vi "Measurement.vi"(0 "Position":T7(array[cluster]) {"Z" format="%.1f"; "Y" format="%.1f"; "X" format="%.1f"}, 1 "setup":T8=enum."Show Setup", 2 "Post Process":T5, 4 "File":T9, 5 "Results file":path, 7 "Raw data file":path, 11 "Setup filename":string) -> (14 "2nd plot":cluster{"Xo":dbl, "Delta X":dbl, dbl[]}[](graph), 19 "Status Out":T4)   [LabVIEW 2010]
uses:
  Anemometry Sub Vis/Controls/Save_Data.ctl
  Anemometry Sub Vis/Controls/Setup.ctl
  Anemometry Sub Vis/Controls/Graph_Type.ctl
  Anemometry Sub Vis/Controls/Post_Process.ctl
  Anemometry Sub Vis/Gen Trav/Multi_Run_Status.ctl
  Anemometry Sub Vis/Controls/Board_Types.ctl
  Anemometry Sub Vis/File/Setup_Filetype.ctl
  Anemometry Sub Vis/Controls/Block_start_and_end.ctl
  ADAM Client/Sub VIs/ADAM Controls/Traverse_Level_State.ctl
  Anemometry Sub Vis/Globals/Trav_pos_global.vi
  Anemometry Sub Vis/Globals/Meas_global.vi
  Anemometry Sub Vis/Acquisition/Data_Translation/DataTranslation_global.vi
  Anemometry Sub Vis/Acquisition/PWA/PWAtasksGLOBAL.vi
  Anemometry Sub Vis/Globals/Preference_global.vi
  Anemometry Sub Vis/Globals/LDA_meas_global_1.vi
  Anemometry Sub Vis/Globals/Dynamic_call_global.ph.vi
  Anemometry Sub Vis/Globals/LDA_meas_global_2.vi
  Anemometry Sub Vis/Globals/Plug_in_data_global.vi
panel:
  in  "PP next block":bool
  out "Pause message":string
  out "Statistics":string[][](table)
  in  "Tab Control":T1(tab)
  out "Measurement time (min)":dbl=6.0 format="%.2f"
  in  "No of bins":i32=80
  in  "Show Smoth":bool=TRUE
  in  "Second Graph":T3={"Plot 1"=2, "Plot 2"=1, "Save graph"=0, "Plot Type"=enum."Vel histogram"} {"Save graph" items=["Do not save plot", "Save plot"]; "Plot 2" items=["Nothing", "Pitot (C)"]; "Plot 1" items=["Nothing", "Pitot (C)"]}
  in  "First Graph":T3={"Plot 1"=1, "Plot 2"=2, "Save graph"=0, "Plot Type"=enum."Velocity trace"} {"Save graph" items=["Do not save plot", "Save plot"]; "Plot 2" items=["Nothing", "Pitot (C)"]; "Plot 1" items=["Nothing", "Pitot (C)"]}
  out "First plot":cluster{"Xo":dbl, "Delta X":dbl, dbl[]}[](graph)
  in  "Comments":string
  out "BSA Diagnostic info":string[][](table)
  out "uv":dbl[][](graph)=[[-0.041806189081711534, -0.046435429052714985, -0.04035660097427599, -0.042187605126076694, -0.042052555599004206]]
  out "u^4":dbl[][](graph)
  out "u^3":dbl[][](graph)
  out "u^2":dbl[][](graph)=[[0.09743628875280319, 0.10575821456272283, 0.10126262927293661, 0.09890442087602569, 0.1022948212436432]]
  out "U":dbl[][](graph)=[[0.8295029456391334, 0.8915896983798417, 0.8415763502225625, 0.8394746126219594, 0.8466062785395404]]
  in  "Block average display control":cluster{"Name":string, "Include":bool}[](array[cluster])=[{"Name"="FF (C)", "Include"=FALSE}]
  out "Array U":dbl[][](array[numeric]) format="%.2e"
  out "Array u^2":dbl[][](array[numeric]) format="%.2e"
  out "Actual Sampling freq":dbl=100.0 format="%.1f"
  in  "Desired Sampling freq (Hz)":dbl=100.0 format="%.1f"
  in  "Correlate?":T6(ring)
  out "Current Block No":i32=5
  in  "Pause":bool
  in  "No of Blocks":i32=5
  in  "stop":bool
  in  "No of samples":i32=1000 min=0 step=1
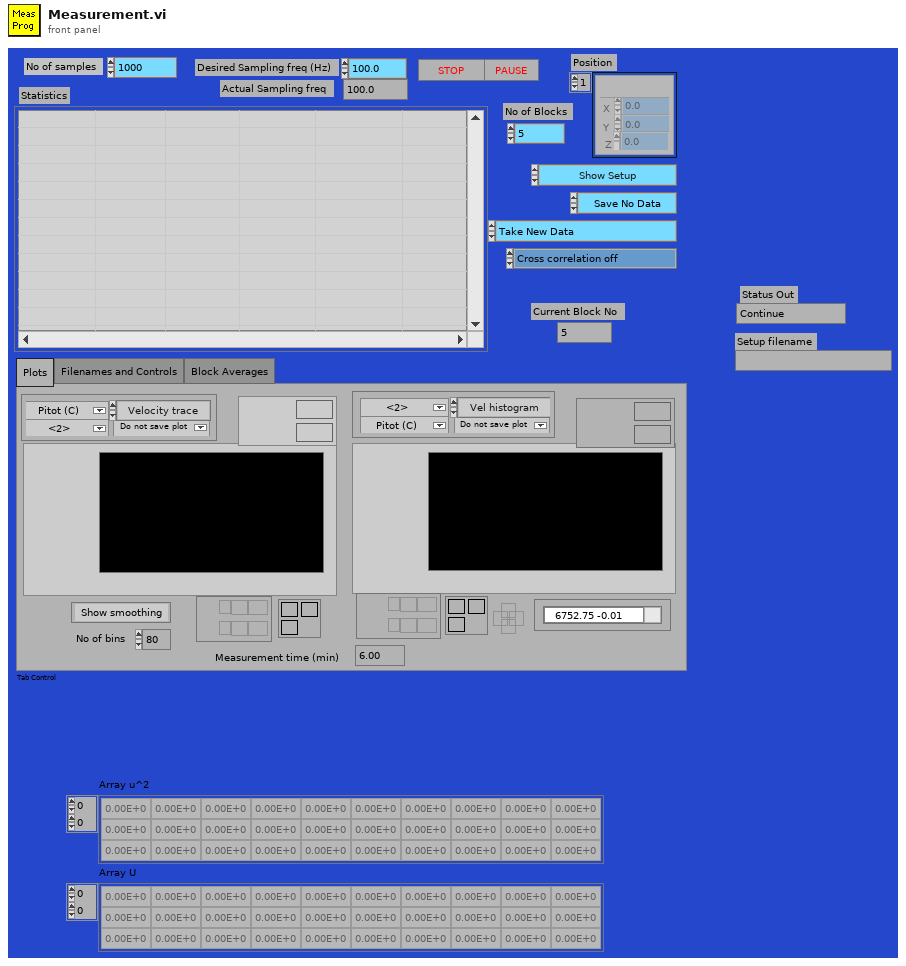
[diagram p1: front panel]
types:
  T1 = enum32{"Plots", "Filenames and Controls", "Block Averages"}
  T2 = typedef "Graph_Type.ctl" = enum16{"Show no graph", "Voltage trace", "Velocity trace", "Vel histogram", "Spectrum", "f.E(f) v Log f", "Auto-Corr"}
  T3 = cluster{"Plot 1":u16, "Plot 2":u16, "Save graph":u16, "Plot Type":T2}
  T4 = typedef "Multi_Run_Status.ctl" = enum16{"Continue", "Jump to Next Point", "Jump to Next Row", "Jump To Fall Back", "Terminate Run"}
  T5 = typedef "Post_Process.ctl" = enum16{"Take New Data", "Post Process Raw Data File"}
  T6 = enum16{"Cross correlation off", "Show correlation panel", "Correlate without activating panel"}
  T7 = cluster{"Name":string, "X":dbl, "Y":dbl, "Z":dbl}[]
  T8 = typedef "Setup.ctl" = enum16{"Run Program", "Show Setup", "Save Current Setup", "Setup Front Panel"}
  T9 = typedef "Save_Data.ctl" = enum16{"Save No Data", "Save Data"}
  T10 = enum32{"Bad", "Idle", "Run top level", "Running"}
  T11 = enum16{"Velocity", "Transit time", "Arrival time"}
  T12 = enum16{"Save no data", "Save data in new files", "Save data in existing files"}
  T13 = typedef "Board_Types.ctl" = enum16{"Simulate", "Local ADAM", "Server ADAM", "NI-DAQmx", "NI-DAQmxBase", "ADC488", "DT LV-link"}
  T14 = typedef "Setup_Filetype.ctl" = enum16{"Measurement Setups", "Calibration Setups", "General", "Results File Plotter Setups", "Speed Calib Tweaks"}
  T15 = typedef "Block_start_and_end.ctl" = cluster{"Started":dbl, "Ended":dbl, "Analogue Frequency Hz":dbl}
  T16 = typedef "Traverse_Level_State.ctl" = enum16{"Running", "Complete"}
  T17 = typedef "Traverse_cluster.ctl" = cluster{"Start X":dbl, "Start Y":dbl, "Start Z":dbl, "End X":dbl, "End Y":dbl, "End Z":dbl, "No. of pts.":i32, "Spacing":T18, "Filename":path, "Tunnel Speed":dbl, "Averaging time (min)":dbl, "Extra Commands":string, "Specific Arguments":string, "Emission Rate (l/min)":dbl, "Trace Gas Concentration (%)":dbl, "Density Ratio":string, "Comments":string, "Row No":i32, "Row Type Selector":T19, "Completion time":string, "Row Duration (mins)":dbl, "No. of Valid pts.":i32, "Meas Setup File":string}
  T18 = typedef "Spacing.ctl" = enum16{"Linear", "Log", "Gauss", "Specified", "N/A"}
  T19 = typedef "Multi_run_mode.ctl" = enum16{"Move Traverse Only", "Set Tunnel Speed Only", "Set Source Only", "Set Measurement Conditions", "Single Measurement", "Vertical Profile", "Lateral Profile", "Longitudinal Profile", "Explore Volume", "Multi-Axis Profile", "Auto Calibrate", "Meas Fast FID Bkgnd", "Check Beam Power", "Scanning Valve Measurement", "Run VI Named:", "Set ADAM Ch", "Wait (minutes)", "Send Message", "Synchronize With:", "Fall Back to this Row", "Turn Off Row Repeating", "Blank Row"}
  T20 = typedef "Analysis_info_cluster.ctl" = cluster{"Colour":u32, "Inst type":T21, "Inst name":string, "Symbol":string, "Code name":string, "Extra Info":string, "Inst Array":T22, "Index":i32, "Voltage Index":i32, "Extra Titles":string[], "Extra Values":string[]}
  T21 = typedef "Inst_type.ctl" = enum16{"Propeller anemometer", "Raw voltage", "Pressure Transducer", "Pitot-static tube", "Preston tube", "Hot wire", "Cross wire 1", "Cross wire 2", "Generic Linear", "Generic Polynomial", "Generic BackPoly", "Fast FID", "Thermocouple", "Cold wire", "Pulsed Wire", "LDA Vel", "LDA Tran time", "LDA Arr time"}
  T22 = typedef "Instrument_Array.ctl" = enum16{"PWA", "LDA", "Analogue"}
  T23 = enum16{"Velocity", "Transit time", "Arrival time"}[]
  T24 = typedef "BSA_Type.ctl" = enum16{"57N11", "BSA F60"}
  T25 = typedef "BSA_info_Cluster.ctl" = cluster{"GPIB Address":string, "No of Check Bytes":i32, "Extra Info":string, "COLOUR":u32, "Wavelength (nm)":dbl}
  T26 = typedef "Ch_and_Spans.ctl" = cluster{"high limit (10V)":sgl, "low limit (-10V)":sgl, "Ch No":i16, "Var name":string, "Use Latest Calib":bool}
  T27 = typedef "Velocity_cluster.ctl" = cluster{"Name":string, "U":dbl, "u^2":dbl, "u^3/(u^2)^(1.5)":dbl, "u^4/(u^2)^2 -3":dbl, "% u'/U":dbl, "Mean % Err":dbl, "u^4":dbl}
  T28 = typedef "Analysis_type_cluster.ctl" = cluster{"Analysis type":T29, "Indicies":i32[], "Name":string, "Inst Array":T22, "Info index":i32}
  T29 = typedef "Analysis_type_Enum.ctl" = enum16{"Slow Response", "Fast Response", "Weighted Fast Response", "Fast FID", "Weighted Fast FID", "Cross Wire", "Weighted Cross Wire", "Weighted LDA"}
  T30 = cluster{"Insts for plotting[0]":u16, "Insts for plotting[1]":u16}
  T31 = typedef "PWA_Data.ctl" = enum16{"No PWA Data", "One Ch PWA"}
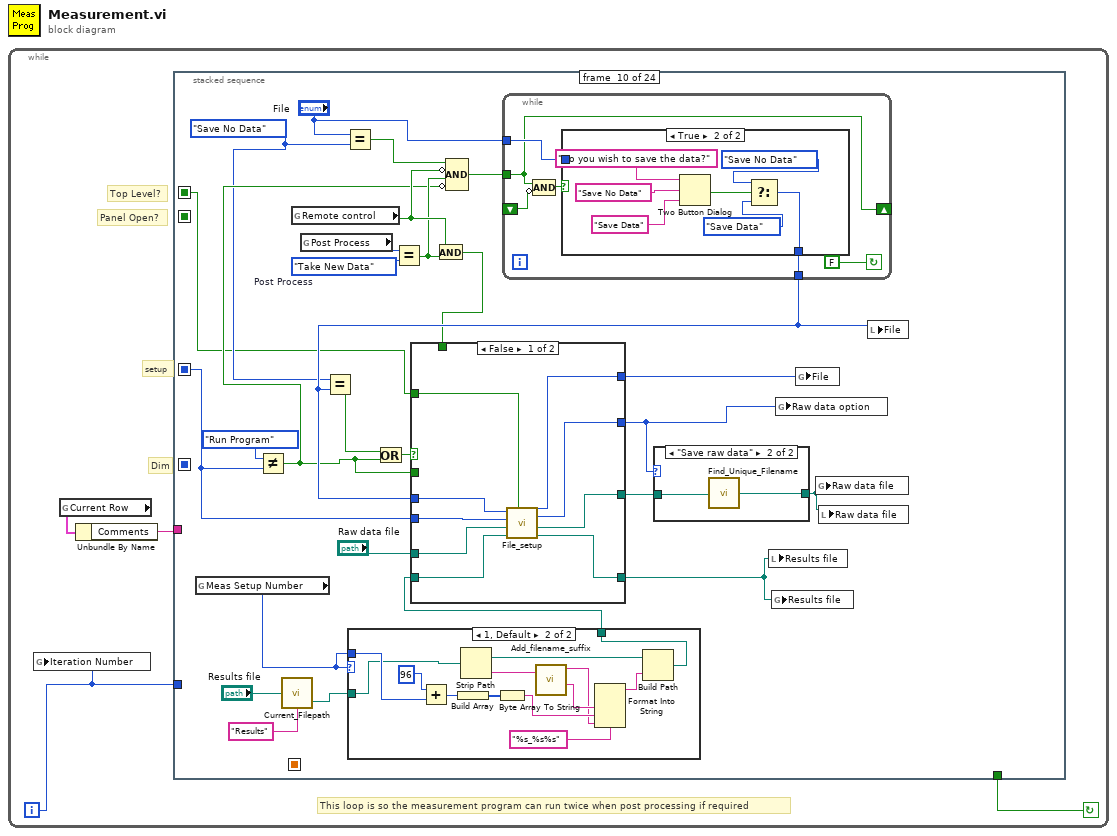
[diagram p0: block diagram]
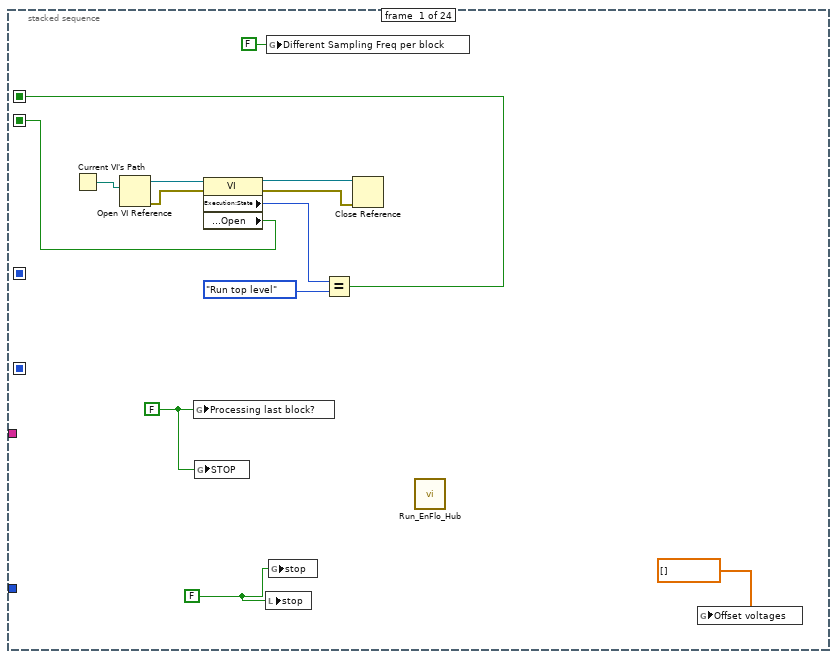
[diagram p2: hidden frame]
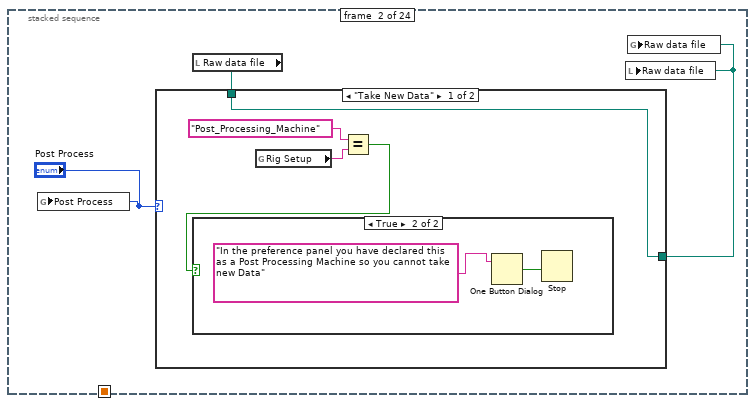
[diagram p3: hidden frame]
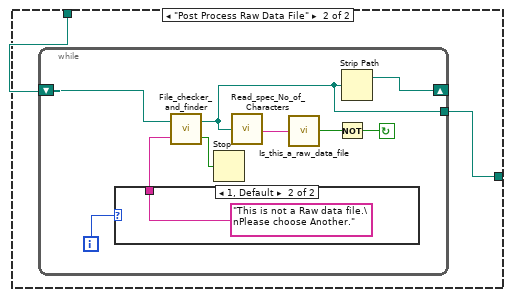
[diagram p5: hidden frame]
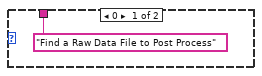
[diagram p6: hidden frame]
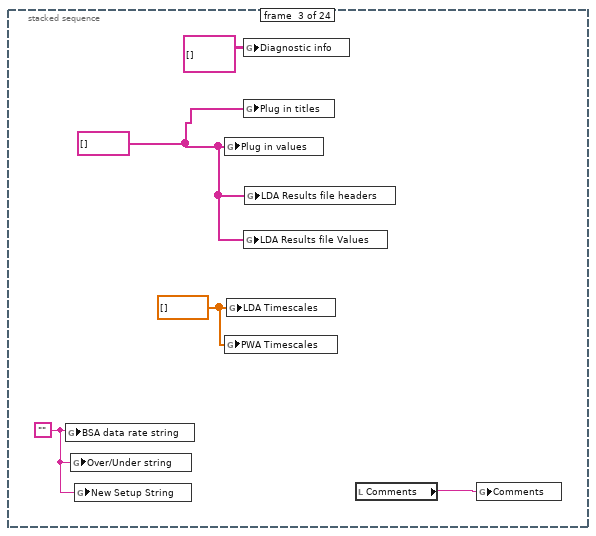
[diagram p7: hidden frame]
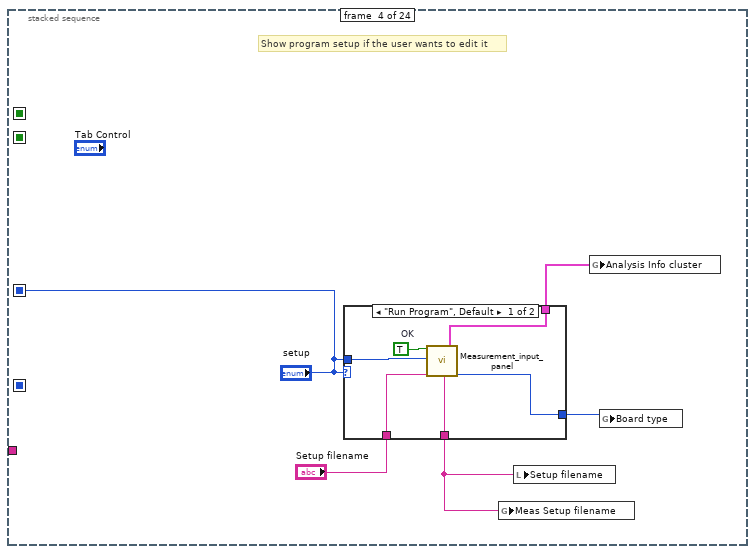
[diagram p8: hidden frame]
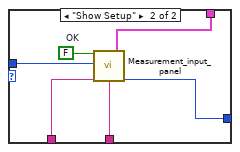
[diagram p9: hidden frame]
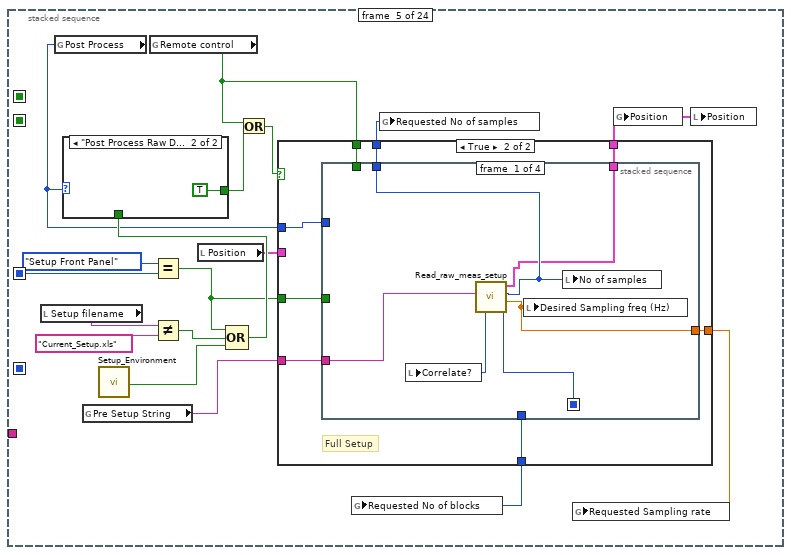
[diagram p10: hidden frame]
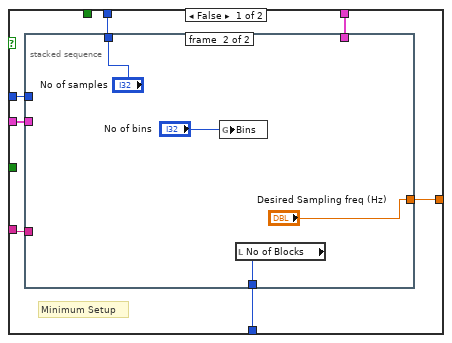
[diagram p12: hidden frame]
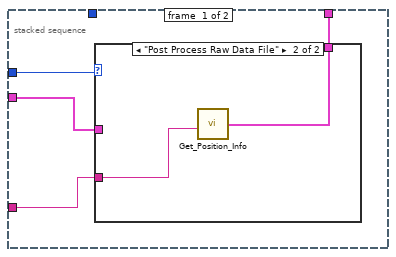
[diagram p13: hidden frame]
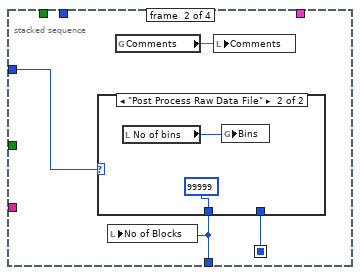
[diagram p15: hidden frame]
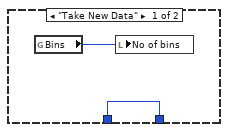
[diagram p16: hidden frame]
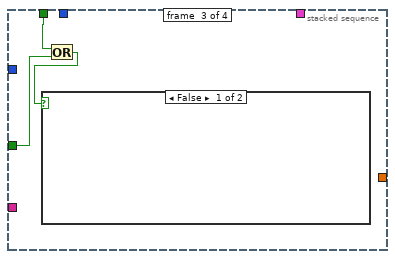
[diagram p17: hidden frame]
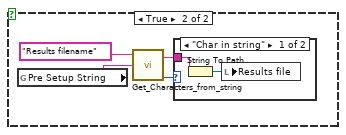
[diagram p18: hidden frame]
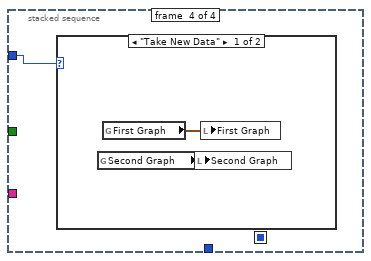
[diagram p20: hidden frame]
diagram:
  n1 = while {
    i -> [w1]
    stop <- w2 continue-if-true
    # "This loop is so the measurement program can run twice when post processing if required"
    # "Panel Open?"
    # "Top Level?"
    # "setup"
    # "Dim"
    n2 = global write "Meas_global.vi" "Iteration Number"(w1) -> ()
    n3 = global read "Trav_pos_global.vi" "Current Row"() -> (w3:T17)
    n4 = Unbundle By Name(w3) -> ("Comments"=w4:string)
    n5 = stacked-sequence {
      seq-local: [_ _ _ _ _ _ _ _ w187 _ _ _ _ _ _ _ _ _ _ _ _ _ _ _] -> [_ _ _ _ _ _ _ _ _ _ _ _ _ _ _ _ _ w624 _ _ _ _ _ _]
      seq-local: [_ _ _ "setup" _ _ _ _ _ _ _ _ _ _ _ _ _ _ _ _ _ _ _ _] -> [_ _ _ _ w71 _ _ _ w179 w264 _ _ _ _ w524 w562 w569 w625 w933 w1009 w1037 _ _ w1112]
      seq-local: [_ _ _ _ _ _ _ _ _ _ _ _ _ _ _ _ w565 _ _ _ _ _ _ _] -> [_ _ _ _ _ _ _ _ _ _ _ _ _ _ _ _ _ w623 w916 _ _ _ _ _]
      seq-local: [w7 _ _ _ _ _ _ _ _ _ _ _ _ _ _ _ _ _ _ _ _ _ _ _] -> [_ _ _ _ _ _ _ _ _ w244 _ _ _ _ w520 _ _ w622 _ _ _ _ _ _]
      seq-local: [w6 _ _ _ _ _ _ _ _ _ _ _ _ _ _ _ _ _ _ _ _ _ _ _] -> [_ _ _ _ _ _ _ _ _ _ _ _ w363 _ _ _ _ _ _ _ _ _ _ _]
      tunnel: w4 -> [_ _ _ _ _ _ _ w172 _ _ _ _ _ _ _ _ _ _ _ _ _ _ w1080 _]
      tunnel: w1 -> [_ _ _ _ _ _ _ _ _ _ _ _ _ _ _ _ _ _ _ _ _ _ w1075 _]
      tunnel: [_ _ _ _ _ _ _ _ _ _ _ _ _ _ _ _ _ _ _ _ _ _ w1074 _] -> w2
      frame #0 {
        w15 = FALSE ("Processing last block?")
        w16 = FALSE ("stop")
        n6 = Current VI's Path() -> (path=w8:path)
        n7 = Open VI Reference(vi path=w8) -> (vi reference=w9:refnum<vi>, error out=w10:errorcluster)  [unwired: 1 in, 4 out]
        n8 = global write "Meas_global.vi" "Processing last block?"(w15) -> ()
        n9 = global write "PWAtasksGLOBAL.vi" "STOP"(w15) -> ()
        n10 = property class="VI"(reference=w9, error in=w10) -> (reference out=w11:refnum<vi>, error out=w12:errorcluster, "Execution:State"=w13:T10, "Front Panel.Open"=w6:bool)
        n11 = local write "stop"(w16) -> ()
        n12 = global write "DataTranslation_global.vi" "Different Sampling Freq per block"(FALSE ("Different Sampling Freq per block")) -> ()
        n13 = global write "Meas_global.vi" "stop"(w16) -> ()
        n14 = Equal?(x=w13, y=T10."Run top level" ("Exec.State")) -> (x = y?=w7:bool)
        n15 = Close Reference(reference=w11, error in (no error)=w12) -> ()  [unwired: 1 out]
        n16 = call "Run_EnFlo_Hub.vi"() -> ()  [unwired: 8 out]
        n17 = global write "Meas_global.vi" "Offset voltages"(dbl[] [] ("Offset voltages used")) -> ()
      }
      frame #1 {
        n18 = global write "Meas_global.vi" "Post Process"("Post Process") -> ()
        n19 = local read "Raw data file"() -> (w20:path)
        n20 = case shown="\"Take New Data\"" "Post Process" {
          tunnel: [w24 w28] -> w19
          tunnel: w20 -> [w24 w27]
          frame "Take New Data" {
            n21 = global read "Preference_global.vi" "Rig Setup"() -> (w23:string)
            n22 = Equal?(x="Post_Processing_Machine" ("Rig Setup"), y=w23) -> (x = y?=w21:bool)
            n23 = case shown="True" w21 {
              frame False {
              }
              frame True {
                n24 = One Button Dialog(message="In the preference panel you have declared this as a Post Processing Machine so you cannot take new Data") -> (true=w25:bool)  [unwired: 1 in]
                n25 = Stop(stop? (T)=w25) -> ()
              }
            }
          }
          frame "Post Process Raw Data File" {
            n26 = while {
              tunnel: [w30] -> w28
              shift-left: w27 -> [w32]
              shift-right: [w31] -> _
              i -> [w33]
              stop <- w34 continue-if-true
              n27 = case shown="1, Default" w33 {
                tunnel: ["Find a Raw Data File to Post Process" ("Promp if not found") "This is not a Raw data file.\nPlease choose Another." ("Promp if not found")] -> w37
                frame 0 {
                }
                frame 1, Default {
                }
              }
              n28 = call "File_checker_and_finder.vi"("Promp if not found"=w37, "Filename In"=w32) -> ("cancelled"=w29:bool, "Filename Out"=w30:path)
              n29 = Stop(stop? (T)=w29) -> ()
              n30 = call "Read_spec_No_of_Characters.vi"("Filename"=w30) -> ("character string"=w36:string)  [unwired: 1 out]
              n31 = call "Is_this_a_raw_data_file.vi"("character string"=w36) -> ("Raw Dat File?"=w35:bool)  [unwired: 2 out]
              n32 = Not(x=w35) -> (.not. x?=w34:bool)
              n33 = Strip Path(path=w30) -> (stripped path=w31:path)  [unwired: 1 out]
            }
          }
        }
        n34 = local write "Raw data file"(w19) -> ()
        n35 = global write "Meas_global.vi" "Raw data file"(w19) -> ()
      }
      frame #2 {
        w42 = dbl[] [] ("LDA Timescales")
        w41 = string[] [] ("Plug in values")
        w44 = ""
        n36 = global write "Meas_global.vi" "BSA data rate string"(w44) -> ()
        n37 = global write "Meas_global.vi" "Over/Under string"(w44) -> ()
        n38 = global write "Meas_global.vi" "New Setup String"(w44) -> ()
        n39 = global write "Dynamic_call_global.ph.vi" "Plug in values"(w41) -> ()
        n40 = global write "PWAtasksGLOBAL.vi" "PWA Timescales"(w42) -> ()
        n41 = global write "LDA_meas_global_1.vi" "LDA Timescales"(w42) -> ()
        n42 = global write "Meas_global.vi" "Diagnostic info"(string[][] [] ("Diagnostic info")) -> ()
        n43 = global write "Dynamic_call_global.ph.vi" "Plug in titles"(w41) -> ()
        n44 = global write "LDA_meas_global_1.vi" "LDA Results file Values"(w41) -> ()
        n45 = global write "LDA_meas_global_1.vi" "LDA Results file headers"(w41) -> ()
        n46 = local read "Comments"() -> (w43:string)
        n47 = global write "Meas_global.vi" "Comments"(w43) -> ()
      }
      frame #3 {
        # "Show program setup if the user wants to edit it"
        n48 = case shown="\"Run Program\", Default" "setup" {
          tunnel: [w54 w60] -> w49
          tunnel: [w53 w59] -> w48
          tunnel: "Setup filename" -> [w52 w58]
          tunnel: [w51 w57] -> w45
          tunnel: "setup" -> [w50 w56]
          frame "Run Program", Default {
            w55 = TRUE  # OK
            n49 = call "Measurement_input_panel.vi"("OK"=w55, "setup"=w50, "Setup filename"=w52) -> ("Setup filename out"=w51:string, "Analysis Info cluster"=w54:T20[], "Board type"=w53:T13)  [unwired: 14 out]
          }
          frame "Show Setup" {
            w61 = FALSE  # OK
            n50 = call "Measurement_input_panel.vi"("OK"=w61, "setup"=w56, "Setup filename"=w58) -> ("Setup filename out"=w57:string, "Analysis Info cluster"=w60:T20[], "Board type"=w59:T13)  [unwired: 14 out]
          }
        }
        n51 = global write "Meas_global.vi" "Meas Setup filename"(w45) -> ()
        n52 = local write "Setup filename"(w45) -> ()
        n53 = global write "Meas_global.vi" "Analysis Info cluster"(w49) -> ()
        n54 = global write "Meas_global.vi" "Board type"(w48) -> ()
      }
      frame #4 {
        n55 = local read "Setup filename"() -> (w75:string)
        n56 = global read "Meas_global.vi" "Post Process"() -> (w70:T5)
        n57 = global read "Meas_global.vi" "Pre Setup String"() -> (w66:string)
        n58 = call "Setup_Environment.vi"() -> ("First Time"=w67:bool)  [unwired: 1 in]
        n59 = global read "Meas_global.vi" "Remote control"() -> (w63:bool)
        n60 = Equal?(x=Setup."Setup Front Panel" ("setup"), y=w71) -> (x = y?=w62:bool)
        n61 = Not Equal?(x=w75, y="Current_Setup.xls" ("Setup filename")) -> (x != y?=w73:bool)
        n62 = local read "Position"() -> (w64:T7)
        n63 = Compound Arithmetic op=OR(w62, w73, w67) -> (w72:bool)
        n64 = case shown="\"Post Process Raw Data File\"" w70 {
          tunnel: [w80 TRUE] -> w79
          tunnel: w72 -> [w80 _]
          frame "Take New Data" {
          }
          frame "Post Process Raw Data File" {
          }
        }
        n65 = Or(x=w63, y=w79) -> (x .or. y?=w78:bool)
        n66 = case shown="True" w78 {
          tunnel: w70 -> [w84 w107]
          tunnel: [w88 w106] -> w68
          tunnel: [w87 w101] -> w77
          tunnel: [w86 w105] -> w76
          tunnel: [w85 w104] -> w65
          tunnel: w66 -> [w83 w103]
          tunnel: w64 -> [w82 _]
          tunnel: w63 -> [_ w102]
          tunnel: w62 -> [_ w100]
          frame False {
            # "Minimum Setup"
            n67 = stacked-sequence {
              tunnel: [_ "Desired Sampling freq (Hz)"] -> w88
              tunnel: [_ w98] -> w87
              tunnel: [_ "No of samples"] -> w86
              tunnel: [w91 _] -> w85
              tunnel: w84 -> [w92 _]
              tunnel: w83 -> [w90 _]
              tunnel: w82 -> [w89 _]
              frame #0 {
                n68 = case shown="\"Post Process Raw Data File\"" w92 {
                  tunnel: [w93 w94] -> w91
                  tunnel: w89 -> [w93 _]
                  tunnel: w90 -> [_ w95]
                  frame "Take New Data" {
                  }
                  frame "Post Process Raw Data File" {
                    n69 = call "Get_Position_Info.vi"("Input string"=w95) -> ("Position"=w94:T7)
                  }
                }
              }
              frame #1 {
                n70 = global write "Meas_global.vi" "Bins"("No of bins") -> ()
                n71 = local read "No of Blocks"() -> (w98:i32)
              }
            }
          }
          frame True {
            # "Full Setup"
            n72 = stacked-sequence {
              seq-local: [w110 _ _ _] -> [_ w115 _ _]
              tunnel: w107 -> [_ w116 _ w131]
              tunnel: [w113 _ _ _] -> w106
              tunnel: [w112 _ _ _] -> w105
              tunnel: [w108 _ _ _] -> w104
              tunnel: w103 -> [w111 _ _ _]
              tunnel: w102 -> [_ _ w124 _]
              tunnel: [_ w114 _ _] -> w101
              tunnel: w100 -> [_ _ w123 _]
              frame #0 {
                n73 = call "Read_raw_meas_setup.vi"("Setup file string"=w111) -> ("No of Blocks"=w110:i32, "Sampling freq (Hz)"=w113:dbl, "No of samples"=w112:i32, "Position"=w108:T7, "Correlate?"=w109:T6)  [unwired: 4 out]
                n74 = local write "Correlate?"(w109) -> ()
                n75 = local write "Desired Sampling freq (Hz)"(w113) -> ()
                n76 = local write "No of samples"(w112) -> ()
              }
              frame #1 {
                n77 = case shown="\"Post Process Raw Data File\"" w116 {
                  tunnel: [w119 99999 ("No of Blocks")] -> w114
                  tunnel: w115 -> [w119 _]
                  frame "Take New Data" {
                    n78 = global read "Meas_global.vi" "Bins"() -> (w118:i32)
                    n79 = local write "No of bins"(w118) -> ()
                  }
                  frame "Post Process Raw Data File" {
                    n80 = local read "No of bins"() -> (w120:i32)
                    n81 = global write "Meas_global.vi" "Bins"(w120) -> ()
                  }
                }
                n82 = local write "No of Blocks"(w114) -> ()
                n83 = global read "Meas_global.vi" "Comments"() -> (w117:string)
                n84 = local write "Comments"(w117) -> ()
              }
              frame #2 {
                n85 = Or(x=w124, y=w123) -> (x .or. y?=w122:bool)
                n86 = case shown="False" w122 {
                  frame False {
                  }
                  frame True {
                    n87 = global read "Meas_global.vi" "Pre Setup String"() -> (w125:string)
                    n88 = call "Get_Characters_from_string.vi"("Input string"=w125, "Variable name"="Results filename") -> ("Status"=w128:enum16{"Char in string", "Char not in string"}, "Value"=w127:string)  [unwired: 1 in]
                    n89 = case shown="\"Char in string\"" w128 {
                      tunnel: w127 -> [w130 _]
                      frame "Char in string" {
                        n90 = String To Path(string=w130) -> (path=w129:path)
                        n91 = local write "Results file"(w129) -> ()
                      }
                      frame "Char not in string" {
                      }
                    }
                  }
                }
              }
              frame #3 {
                n92 = case shown="\"Take New Data\"" w131 {
                  frame "Take New Data" {
                    n93 = global read "Meas_global.vi" "Second Graph"() -> (w132:T3)
                    n94 = global read "Meas_global.vi" "First Graph"() -> (w133:T3)
                    n95 = local write "Second Graph"(w132) -> ()
                    n96 = local write "First Graph"(w133) -> ()
                  }
                  frame "Post Process Raw Data File" {
                  }
                }
              }
            }
          }
        }
        n97 = global write "Meas_global.vi" "Requested No of blocks"(w77) -> ()
        n98 = global write "Meas_global.vi" "Requested No of samples"(w76) -> ()
        n99 = global write "Meas_global.vi" "Requested Sampling rate"(w68) -> ()
        n100 = global write "Meas_global.vi" "Position"(w65) -> ()
        n101 = local write "Position"(w65) -> ()
      }
      frame #5 {
        n102 = global read "Meas_global.vi" "Post Process"() -> (w134:T5)
        n103 = case shown="\"Post Process Raw Data File\"" w134 {
          tunnel: [w137 w138] -> w135
          frame "Take New Data" {
            n104 = Get Date/Time In Seconds() -> (seconds since 1Jan1904=w136:timestamp)
            n105 = To Double Precision Float(number=w136) -> (double precision float=w137:dbl)
          }
          frame "Post Process Raw Data File" {
            n106 = global read "Meas_global.vi" "Pre Setup String"() -> (w141:string)
            n107 = call "Get_Characters_from_string.vi"("Input string"=w141, "Variable name"="Seconds since 1/1/04") -> ("Value"=w139:string)  [unwired: 1 in, 1 out]
            n108 = call "String_2_Number.vi"("Value"=w139) -> ("Numeric"=w138:dbl)
          }
        }
        n109 = global write "Meas_global.vi" "Time Data was Aquired"(w135) -> ()
      }
      frame #6 {
        n110 = global read "Dynamic_call_global.ph.vi" "Initial Plug Ins"() -> (w143:string[])
        n111 = global read "Dynamic_call_global.ph.vi" "Initial Plug Ins Extra"() -> (w144:string[])
        n112 = Build Array (concatenate)(w144, w143) -> (w142:string[])
        n113 = Array Size(array=w142) -> (size(s)=w146:i32)
        n114 = Greater Than 0?(x=w146) -> (x > 0?=w145:bool)
        n115 = case shown="True" w145 {
          tunnel: w142 -> [_ w147]
          frame False {
          }
          frame True {
            n116 = stacked-sequence {
              tunnel: w147 -> [w149 _]
              frame #0 {
                n117 = global read "Meas_global.vi" "Post Process"() -> (w151:T5)
                n118 = call "Plug_in_Directories.vi"() -> ("Initial"=w148:path)  [unwired: 3 out]
                n119 = Equal?(x=w151, y=Post_Process."Post Process Raw Data File" ("Post Process")) -> (x = y?=w150:bool)
                n120 = for {
                  tunnel: w150 -> [w157]
                  tunnel: w149 -> [w154] mode=indexing
                  tunnel: w148 -> [w153]
                  w164 = FALSE  # Dialog Box (T)
                  n121 = Build Path(base path=w153, name or relative path=w154) -> (appended path=w155:path)
                  n122 = Open VI Reference(vi path=w155) -> (vi reference=w162:refnum<vi>, error out=w161:errorcluster)  [unwired: 2 in, 3 out]
                  n123 = property class="VI"(reference=w162, error in=w161, "Front Panel Window:Open"=TRUE ("Wait until done")) -> (reference out=w160:refnum<vi>, error out=w159:errorcluster)
                  n124 = invoke class="VI" method="Run VI"(reference=w160, error in=w159, "Wait until done"=w157, "Auto Dispose Ref"=FALSE) -> (reference out=w167:refnum<vi>, error out=w166:errorcluster)  [unwired: 1 in, 3 out]
                  n125 = Close Reference(reference=w167, error in (no error)=w166) -> (error out=w165:errorcluster)
                  n126 = call "EnFlo_Error_Handler.vi"("error in (no error)"=w165, "Error Type"="Launching Initial Plug In", "Dialog Box (T)"=w164) -> ()  [unwired: 3 out]
                }
              }
              frame #1 {
                n127 = global read "Meas_global.vi" "Requested No of blocks"() -> (w169:i32)
                n128 = global read "Meas_global.vi" "Comments"() -> (w168:string)
                n129 = local write "Comments"(w168) -> ()
                n130 = local write "No of Blocks"(w169) -> ()
              }
            }
          }
        }
      }
      frame #7 {
        n131 = local read "Comments"() -> (w173:string)
        n132 = Concatenate Strings(w172, w173) -> (w171:string)
        n133 = call "Text_without_format.vi"("Input string"=w171) -> ("Output string"=w170:string)
        n134 = local write "Comments"(w170) -> ()
        n135 = global write "Meas_global.vi" "Comments"(w170) -> ()
      }
      frame #8 {
        n136 = global read "Meas_global.vi" "dimensions"() -> (w187:enum16{"1D", "2D"})
        n137 = global read "Meas_global.vi" "Post Process"() -> (w186:T5)
        n138 = global read "Meas_global.vi" "LDA data"() -> (w184:enum16{"No LDA data", "Take LDA data"})
        n139 = Equal?(x=Setup."Run Program" ("setup"), y=w179) -> (x = y?=w182:bool)
        n140 = Equal?(x=w179, y=Setup."Show Setup" ("setup")) -> (x = y?=w174:bool)
        n141 = Equal?(x=w184, y=enum16{"No LDA data", "Take LDA data"}."Take LDA data" ("LDA data")) -> (x = y?=w177:bool)
        n142 = Or(x=w182, y=w174) -> (x .or. y?=w176:bool)
        n143 = Equal?(x=w186, y=Post_Process."Take New Data" ("Post Process")) -> (x = y?=w178:bool)
        n144 = Compound Arithmetic op=AND(w176, w177, w178) -> (w175:bool)
        n145 = case shown="True" w175 {
          tunnel: w187 -> [_ w196]
          tunnel: w179 -> [_ w195]
          tunnel: w174 -> [_ w193]
          frame False {
            n146 = global write "LDA_meas_global_1.vi" "Number of measured quantities"(3 ("Number of measured quantities")) -> ()
            n147 = Build Array(T11."Velocity", T11."Transit time", T11."Arrival time") -> (w188:T23)
            n148 = global write "LDA_meas_global_2.vi" "data type"(w188) -> ()
            n149 = global write "LDA_meas_global_1.vi" "data type"(w188) -> ()
          }
          frame True {
            n150 = global read "LDA_meas_global_1.vi" "BSA Type"() -> (w194:T24)
            n151 = case shown="\"BSA F60\"" w194 {
              tunnel: w196 -> [w198 _]
              tunnel: w195 -> [w197 _]
              tunnel: w193 -> [_ w234]
              frame "57N11" {
                n152 = stacked-sequence {
                  tunnel: w198 -> [w201 w227]
                  tunnel: w197 -> [w200 _]
                  frame #0 {
                    n153 = global read "Meas_global.vi" "Remote control"() -> (w199:bool)
                    n154 = case shown="\"2D\"" w201 {
                      tunnel: w200 -> [w203 w216]
                      tunnel: w199 -> [w202 w215]
                      frame "2D" {
                        n155 = while {
                          tunnel: w202 -> [w204]
                          tunnel: w203 -> [w205]
                          stop <- w206 continue-if-true
                          n156 = stacked-sequence {
                            tunnel: [_ _ w212] -> w206
                            tunnel: w205 -> [w207 w209 _]
                            tunnel: w204 -> [_ _ w211]
                            frame #0 {
                              w208 = "1"  # BSA Number
                              n157 = call "Control_BSA_setup.vi"("setup"=w207, "BSA number"=w208) -> ()  [unwired: 14 out]
                            }
                            frame #1 {
                              w210 = "2"  # BSA Number
                              n158 = call "Control_BSA_setup.vi"("setup"=w209, "BSA number"=w210) -> ()  [unwired: 14 out]
                            }
                            frame #2 {
                              n159 = case shown="False" w211 {
                                tunnel: [w213 FALSE ("ok")] -> w212
                                frame False {
                                n160 = call "BSA_setup_check.vi"() -> ("ok"=w213:bool)
                                }
                                frame True {
                                }
                              }
                            }
                          }
                        }
                      }
                      frame "1D" {
                        n161 = stacked-sequence {
                          tunnel: w216 -> [w217 _]
                          tunnel: w215 -> [_ _]
                          frame #0 {
                            w218 = "1"  # BSA Number
                            n162 = call "Control_BSA_setup.vi"("setup"=w217, "BSA number"=w218) -> ()  [unwired: 14 out]
                          }
                          frame #1 {
                            n163 = global read "LDA_meas_global_2.vi" "BSA2 info"() -> (w219:T25)
                            n164 = Unbundle By Name(w219) -> ("GPIB Address"=w220:string)
                            n165 = call "Set_BSA_Coincidence.vi"("GPIB address"=w220, "Set Coincidence"=enum16{"Slave", "Master", "Private"}."Slave") -> ()  [unwired: 1 in, 5 out]
                          }
                        }
                      }
                    }
                  }
                  frame #1 {
                    n166 = global read "Meas_global.vi" "Remote control"() -> (w225:bool)
                    n167 = Equal?(x=w227, y=enum16{"1D", "2D"}."2D" ("dimensions")) -> (x = y?=w223:bool)
                    n168 = Not(x=w225) -> (.not. x?=w224:bool)
                    n169 = And(x=w224, y=w223) -> (x .and. y?=w222:bool)
                    n170 = case shown="True" w222 {
                      frame False {
                      }
                      frame True {
                        n171 = global read "LDA_meas_global_1.vi" "BSA1 info"() -> (w229:T25)
                        n172 = global read "LDA_meas_global_2.vi" "BSA2 info"() -> (w230:T25)
                        n173 = Build Array(w229, w230) -> (w228:T25[])
                        n174 = for {
                          tunnel: w228 -> [w232] mode=indexing
                          n175 = Unbundle By Name(w232) -> ("GPIB Address"=w231:string)
                          n176 = call "Set_BSA_Coincidence.vi"("GPIB address"=w231, "Set Coincidence"=enum16{"Slave", "Master", "Private"}."Master") -> ()  [unwired: 1 in, 5 out]
                        }
                      }
                    }
                  }
                }
              }
              frame "BSA F60" {
                n177 = disable-structure shown="TARGET_TYPE==Windows" {
                  disable-tunnel: w234 -> [_ w235]
                  frame condition #0 {
                  }
                  frame condition #1 (active) {
                    n178 = while {
                      tunnel: w235 -> [w238]
                      stop <- w236 continue-if-true
                      n179 = call "Edit_BSA_IP.vi"("Show Panel"=w238) -> ("Run LDA Diagnostic Out"=w237:bool)  [unwired: 2 out]
                      n180 = case shown="False" w237 {
                        tunnel: [FALSE w240] -> w236
                        frame False {
                        }
                        frame True {
                          n181 = call "F60_Diagnostic.vi"() -> ("Edit BSA Setup Out"=w240:bool)  [unwired: 11 in]
                        }
                      }
                    }
                  }
                }
              }
            }
          }
        }
      }
      frame #9 {
        w249 = Save_Data."Save No Data" ("File")
        w265 = Post_Process."Take New Data"  # Post Process
        n182 = global read "Trav_pos_global.vi" "Meas Setup Number"() -> (w245:i32)
        n183 = Not Equal?(x=Setup."Run Program" ("setup"), y=w264) -> (x != y?=w250:bool)
        n184 = call "Current_Filepath.vi"("Filename in"="Results file", "Data Type"="Results") -> ("Filename Out"=w243:path)  [unwired: 1 out]
        n185 = global read "Meas_global.vi" "Remote control"() -> (w261:bool)
        n186 = global read "Meas_global.vi" "Post Process"() -> (w252:T5)
        n187 = Equal?(x="File", y=w249) -> (x = y?=w259:bool)
        n188 = case shown="1, Default" w245 {
          tunnel: [w268 w270] -> w246
          tunnel: w243 -> [w268 w277]
          tunnel: w245 -> [_ w278]
          frame 0 {
          }
          frame 1, Default {
            n189 = Add(x=96, y=w278) -> (x+y=w280:i32)
            n190 = Build Array(w280) -> (w281:i32[])
            n191 = Strip Path(path=w277) -> (stripped path=w271:path, name=w276:string)
            n192 = Byte Array To String(unsigned byte array=w281) -> (string=w274:string)
            n193 = call "Add_filename_suffix.vi"("Filename"=w276) -> ("Original Suffix"=w273:string, "Base name"=w275:string)  [unwired: 1 in, 2 out]
            n194 = Format Into String(format string="%s_%s%s", w275, w274, w273) -> (resulting string=w272:string)  [unwired: 2 in, 1 out]
            n195 = Build Path(base path=w271, name or relative path=w272) -> (appended path=w270:path)
          }
        }
        n196 = Equal?(x=w252, y=w265) -> (x = y?=w251:bool)
        n197 = And(x=w261, y=w251) -> (x .and. y?=w257:bool)
        n198 = Compound Arithmetic op=AND(w259, invert w261, w251, invert w250) -> (w260:bool)
        n199 = while {
          shift-left: _ -> [w286]
          shift-right: [w283] -> _
          tunnel: "File" -> [w284]
          tunnel: [w287] -> w258
          tunnel: w260 -> [w283]
          stop <- FALSE continue-if-true
          n200 = Compound Arithmetic op=AND(w283, invert w286) -> (w285:bool)
          n201 = case shown="True" w285 {
            tunnel: [w288 w291] -> w287
            tunnel: w284 -> [w288 _]
            frame False {
            }
            frame True {
              n202 = Two Button Dialog(message="Do you wish to save the data?", 1:"Save Data" ("F button name (\"Cancel\")"), 2:"Save No Data" ("T button name (\"OK\")")) -> (T button?=w292:bool)
              n203 = Select(t=Save_Data."Save No Data" ("File"), s=w292, f=Save_Data."Save Data" ("File")) -> (s? t:f=w291:T9)
            }
          }
        }
        n204 = Equal?(x=w249, y=w258) -> (x = y?=w248:bool)
        n205 = Or(x=w248, y=w250) -> (x .or. y?=w263:bool)
        n206 = case shown="False" w263 {
          tunnel: w246 -> [w307 w315]
          tunnel: [w306 w315] -> w266
          tunnel: "Raw data file" -> [w305 w316]
          tunnel: [w300 w316] -> w255
          tunnel: w264 -> [w304 _]
          tunnel: w258 -> [w303 _]
          tunnel: [w301 T12."Save no data" ("File output")] -> w253
          tunnel: [w302 w313] -> w247
          tunnel: w257 -> [_ w310]
          tunnel: w250 -> [_ w309]
          tunnel: w244 -> [w299 _]
          frame False {
            n207 = call "File_setup.vi"("Measurement is top level?"=w299, "Results file"=w307, "Raw data file"=w305, "setup"=w304, "File"=w303) -> ("Results file output"=w306:path, "Raw data file output"=w300:path, "Raw data option"=w302:enum16{"Save raw data", "Raw data not saved"}, "File output"=w301:T12)
          }
          frame True {
            w311 = enum16{"Save raw data", "Raw data not saved"}."Raw data not saved"  # Raw data option
            n208 = global read "Meas_global.vi" "Raw data option"() -> (w312:enum16{"Save raw data", "Raw data not saved"})
            n209 = Compound Arithmetic op=AND(w310, invert w309) -> (w308:bool)
            n210 = Select(t=w312, s=w308, f=w311) -> (s? t:f=w313:enum16{"Save raw data", "Raw data not saved"})
          }
        }
        n211 = case shown="\"Save raw data\"" w247 {
          tunnel: w255 -> [w296 w298]
          tunnel: [w296 w297] -> w254
          frame "Raw data not saved" {
          }
          frame "Save raw data" {
            n212 = call "Find_Unique_Filename.vi"("Path In"=w298) -> ("Unique Path Out"=w297:path)  [unwired: 1 in, 1 out]
          }
        }
        n213 = local write "Results file"(w266) -> ()
        n214 = global write "Meas_global.vi" "Results file"(w266) -> ()
        n215 = global write "Meas_global.vi" "Raw data option"(w247) -> ()
        n216 = global write "Meas_global.vi" "File"(w253) -> ()
        n217 = global write "Meas_global.vi" "Raw data file"(w254) -> ()
        n218 = local write "Raw data file"(w254) -> ()
        n219 = local write "File"(w258) -> ()
      }
      frame #10 {
        n220 = global read "Meas_global.vi" "Ch & spans"() -> (w317:T26[])
        n221 = local read "Block average display control"() -> (w322:cluster{"Name":string, "Include":bool}[])
        n222 = global read "Meas_global.vi" "Velocity Cluster Array"() -> (w321:T27[])
        n223 = global write "Meas_global.vi" "Ch & spans + mod limits"(w317) -> ()
        n224 = global read "Meas_global.vi" "Analysis Info cluster"() -> (w327:T20[])
        n225 = call "Determine_Meas_Analysis.vi"("Analogue Channels"=w327) -> ("Analysis Info Cluster"=w324:T20[], "Analysis Type Array"=w326:T28[])
        n226 = for {
          tunnel: w324 -> [w337] mode=indexing
          tunnel: w322 -> [w336]
          tunnel: w321 -> [w334]
          tunnel: [w328] -> w320 mode=indexing
          tunnel: [w331] -> w319 mode=indexing
          tunnel: [w330] -> w318 mode=indexing
          i -> [w335]
          w329 = nan ("Mean % Err")
          n227 = Unbundle By Name(w337) -> ("Inst name"=w328:string)
          n228 = Index Array(array=w334, index=w335) -> (element=w333:T27)
          n229 = Index Array(array=w336, index=w335) -> (element=w332:cluster{"Name":string, "Include":bool})
          n230 = Bundle By Name(cluster=w332, "Name"=w328) -> (w331:cluster{"Name":string, "Include":bool})
          n231 = Bundle By Name(cluster=w333, "Name"=w328, "Mean % Err"=w329, "% u'/U"=w329) -> (w330:T27)
        }
        n232 = Build Array (concatenate)("Nothing", w320) -> (w323:string[])
        n233 = local write "Block average display control"(w319) -> ()
        n234 = global write "Meas_global.vi" "Analysis type array"(w326) -> ()
        n235 = global write "Meas_global.vi" "Analysis Info cluster"(w324) -> ()
        n236 = global write "Meas_global.vi" "Velocity Cluster Array"(w318) -> ()
        n237 = property on="Plot 1" class="Ring (strict)"("Strings []"=w323) -> ()  [unwired: 2 in, 2 out]
        n238 = property on="Plot 1" class="Ring (strict)"("Strings []"=w323) -> ()  [unwired: 2 in, 2 out]
        n239 = property on="Plot 2" class="Ring (strict)"("Strings []"=w323) -> ()  [unwired: 2 in, 2 out]
        n240 = property on="Plot 2" class="Ring (strict)"("Strings []"=w323) -> ()  [unwired: 2 in, 2 out]
      }
      frame #11 {
        n241 = global read "Meas_global.vi" "Analysis Info cluster"() -> (w350:T20[])
        n242 = for {
          tunnel: w350 -> [w354] mode=indexing
          tunnel: [w353] -> w349 mode=indexing
          tunnel: [w352] -> w340
          i -> [w352]
          n243 = Unbundle By Name(w354) -> ("Inst name"=w353:string)
        }
        n244 = Greater Than 0?(x=w340) -> (x > 0?=w339:bool)
        n245 = Select(t="Correlate?", s=w339, f=T6."Cross correlation off" ("Correlate?")) -> (s? t:f=w341:T6)
        n246 = case shown="\"Correlate without activating panel\"" w341 {
          tunnel: w349 -> [_ w359 w361]
          tunnel: [w356 w358 w360] -> w338
          frame "Cross correlation off" {
            n247 = Initialize Array(0) -> (w356:i32[][])  [unwired: 2 out]
          }
          frame "Show correlation panel" {
            w357 = FALSE  # OK
            n248 = call "Correlation_Display.vi"("Inst names"=w359, "OK"=w357) -> ("correlation array"=w358:i32[][])  [unwired: 2 in, 2 out]
          }
          frame "Correlate without activating panel" {
            n249 = call "Correlation_Display.vi"("Inst names"=w361, "OK"=TRUE) -> ("correlation array"=w360:i32[][])  [unwired: 2 in, 2 out]
          }
        }
        n250 = global read "Meas_global.vi" "Position"() -> (w348:T7)
        n251 = local write "Position"(w348) -> ()
        n252 = global write "Meas_global.vi" "correlate"(w338) -> ()
        n253 = Array Size(array=w338) -> (size(s)=w347:i32[])
        n254 = Index Array(array=w347, index=0) -> (element=w345:i32)
        n255 = Equal To 0?(x=w345) -> (x = 0?=w344:bool)
        n256 = case shown="True" w344 {
          frame False {
          }
          frame True {
            n257 = local write "Correlate?"(T6."Cross correlation off" ("Correlate?")) -> ()
          }
        }
      }
      frame #12 {
        n258 = stacked-sequence {
          seq-local: [w369 _] -> [_ w391]
          tunnel: w363 -> [w368 _]
          frame #0 {
            n259 = call "LDA+_An_Analysis_mode.vi"("Second Graph"="Second Graph", "First Graph"="First Graph") -> ("Second Graph out"=w364:T3, "First Graph out"=w366:T3)  [unwired: 6 out]
            n260 = case shown="False" w368 {
              tunnel: [w379 w390] -> w367
              tunnel: w366 -> [w378 w390]
              tunnel: [w377 w389] -> w365
              tunnel: w364 -> [w376 w389]
              frame False {
                w374 = Graph_Type."Show no graph" ("Plot Type")
                n261 = Unbundle By Name(w378) -> ("Save graph"=w380:u16)
                n262 = Unbundle By Name(w376) -> ("Save graph"=w375:u16)
                n263 = case shown="0, Default" w380 {
                  tunnel: [w386 w388] -> w379
                  tunnel: w378 -> [w387 w388]
                  tunnel: w374 -> [w385 _]
                  frame 0, Default {
                    n264 = Bundle By Name(cluster=w387, "Plot Type"=w385) -> (w386:T3)
                  }
                  frame 1 {
                  }
                }
                n265 = case shown="0, Default" w375 {
                  tunnel: [w382 w384] -> w377
                  tunnel: w376 -> [w383 w384]
                  tunnel: w374 -> [w381 _]
                  frame 0, Default {
                    n266 = Bundle By Name(cluster=w383, "Plot Type"=w381) -> (w382:T3)
                  }
                  frame 1 {
                  }
                }
              }
              frame True {
              }
            }
            n267 = local write "Second Graph"(w365) -> ()
            n268 = local write "First Graph"(w367) -> ()
            n269 = global write "Meas_global.vi" "Second Graph"(w365) -> ()
            n270 = global write "Meas_global.vi" "First Graph"(w367) -> ()
            n271 = Unbundle By Name(w365) -> ("Plot Type"=w373:T2)
            n272 = Unbundle By Name(w367) -> ("Plot Type"=w372:T2)
            n273 = Build Array(w372, w373) -> (w369:T2[])
          }
          frame #1 {
            n274 = global read "Meas_global.vi" "Insts for plotting"() -> (w392:u16[][])
            n275 = for {
              tunnel: w392 -> [w394] mode=indexing
              tunnel: w391 -> [w393] mode=indexing
              i -> [w395]
              n276 = stacked-sequence {
                seq-local: [w398 _] -> [_ w408]
                seq-local: [w399 _] -> [_ w407]
                tunnel: w395 -> [_ w411]
                tunnel: w394 -> [w397 _]
                tunnel: w393 -> [_ w403]
                frame #0 {
                  n277 = property on="Plot 1" class="Ring (strict)"() -> ("Strings []"=w396:string[])  [unwired: 2 in, 2 out]
                  n278 = Array To Cluster(array=w397) -> (cluster=w402:T30)
                  n279 = Unbundle(w402) -> ("Insts for plotting[0]"=w401:u16, "Insts for plotting[1]"=w400:u16)
                  n280 = Index Array(array=w396, index=w401) -> (element=w398:string)
                  n281 = Index Array(array=w396, index=w400) -> (element=w399:string)
                }
                frame #1 {
                  n282 = case shown="\"Auto-Corr\"" w403 {
                    tunnel: [u8 0 u8 0 u8 0 u8 0 u8 0 u8 1 u8 0] -> w415
                    tunnel: [u8 0 u8 0 u8 0 u8 0 u8 1 u8 1 u8 0] -> w414
                    tunnel: [u8 0 u8 0 u8 0 u8 0 u8 1 u8 1 u8 0] -> w413
                    tunnel: [u8 0 u8 0 u8 0 u8 0 u8 1 u8 0 u8 0] -> w412
                    tunnel: [FALSE TRUE TRUE TRUE TRUE TRUE TRUE] -> w406
                    tunnel: [u8 0 u8 0 u8 0 u8 2 u8 0 u8 0 u8 2] -> w405
                    tunnel: [u8 0 u8 4 u8 1 u8 2 u8 0 u8 0 u8 1] -> w404
                    frame "Show no graph" {
                    }
                    frame "Voltage trace" {
                    }
                    frame "Velocity trace" {
                    }
                    frame "Vel histogram" {
                    }
                    frame "Spectrum" {
                    }
                    frame "f.E(f) v Log f" {
                    }
                    frame "Auto-Corr" {
                    }
                  }
                  n283 = case shown="0, Default" w411 {
                    tunnel: w406 -> [w426 w437]
                    tunnel: w415 -> [w425 w436]
                    tunnel: w414 -> [w424 w435]
                    tunnel: w413 -> [w423 w434]
                    tunnel: w412 -> [w422 w433]
                    tunnel: u32 0 -> [w421 w432]
                    tunnel: u32 1 -> [w420 w430]
                    tunnel: w408 -> [w419 w431]
                    tunnel: w407 -> [w418 w429]
                    tunnel: w405 -> [w417 w428]
                    tunnel: w404 -> [w416 w427]
                    frame 0, Default {
                      n284 = property on="First plot" class="WFGraph (strict)"("Visible"=w426, "X Scale.Format & Precision:Format"=w425, "X Scale.Mapping Mode"=w424, "Y Scale.Format & Precision:Format"=w423, "Y Scale.Mapping Mode"=w422, "Active Plot"=w421, "Plot.Plot Name"=w419, "Active Plot"=w420, "Plot.Plot Name"=w418, "X Scale.Format & Precision:Precision"=w417, "Y Scale.Format & Precision:Precision"=w416) -> ()  [unwired: 2 in, 2 out]
                    }
                    frame 1 {
                      n285 = property on="2nd plot" class="WFGraph (strict)"("Visible"=w437, "X Scale.Format & Precision:Format"=w436, "X Scale.Mapping Mode"=w435, "Y Scale.Format & Precision:Format"=w434, "Y Scale.Mapping Mode"=w433, "Active Plot"=w432, "Plot.Plot Name"=w431, "Active Plot"=w430, "Plot.Plot Name"=w429, "X Scale.Format & Precision:Precision"=w428, "Y Scale.Format & Precision:Precision"=w427) -> ()  [unwired: 2 in, 2 out]
                    }
                  }
                }
              }
            }
          }
        }
      }
      frame #13 {
        n286 = local read "Second Graph"() -> (w498:T3)
        n287 = local read "First Graph"() -> (w497:T3)
        n288 = Unbundle By Name(w497) -> ("Plot 1"=w490:u16, "Plot 2"=w491:u16)
        n289 = Unbundle By Name(w498) -> ("Plot 1"=w492:u16, "Plot 2"=w493:u16)
        n290 = Build Array(w490, w491) -> (w494:u16[])
        n291 = Build Array(w492, w493) -> (w495:u16[])
        n292 = global read "Meas_global.vi" "Analysis Info cluster"() -> (w499:T20[])
        n293 = Decrement(x=w494) -> (x-1=w488:u16[])
        n294 = Decrement(x=w495) -> (x-1=w496:u16[])
        n295 = for {
          tunnel: w499 -> [w507]
          tunnel: w488 -> [w506] mode=indexing
          shift-right: [w500] -> _
          shift-left: u32 0 -> [w502]
          i -> [w501]
          n296 = Index Array(array=w507, index=w506) -> (element=w508:T20)
          n297 = Unbundle By Name(w508) -> ("Colour"=w503:u32)
          n298 = Equal?(x=w503, y=w502) -> (x = y?=w505:bool)
          n299 = Select(t=u32 13434624, s=w505, f=w503) -> (s? t:f=w500:u32)
          n300 = property on="First plot" class="WFGraph (strict)"("Active Plot"=w501, "Plot.Plot Color"=w500, "Plot.Fill/Point Color"=w500) -> ()  [unwired: 2 in, 2 out]
        }
        n301 = for {
          tunnel: w499 -> [w516]
          tunnel: w496 -> [w515] mode=indexing
          shift-right: [w511] -> _
          shift-left: u32 0 -> [w509]
          i -> [w514]
          n302 = Index Array(array=w516, index=w515) -> (element=w517:T20)
          n303 = Unbundle By Name(w517) -> ("Colour"=w510:u32)
          n304 = Equal?(x=w510, y=w509) -> (x = y?=w513:bool)
          n305 = Select(t=u32 13434624, s=w513, f=w510) -> (s? t:f=w511:u32)
          n306 = property on="2nd plot" class="WFGraph (strict)"("Active Plot"=w514, "Plot.Plot Color"=w511, "Plot.Fill/Point Color"=w511) -> ()  [unwired: 2 in, 2 out]
        }
      }
      frame #14 {
        n307 = global read "DataTranslation_global.vi" "Different Sampling Freq per block"() -> (w518:bool)
        n308 = global read "Meas_global.vi" "Remote control"() -> (w527:bool)
        n309 = global read "Meas_global.vi" "Post Process"() -> (w530:T5)
        n310 = global read "Meas_global.vi" "PWA Data"() -> (w519:T31)
        n311 = case shown="\"One Ch PWA\"" w519 {
          tunnel: [w531 w536] -> w521
          frame "No PWA Data" {
            n312 = local read "Desired Sampling freq (Hz)"() -> (w533:dbl)
            n313 = local read "No of samples"() -> (w532:i32)
            n314 = Divide(x=w532, y=w533) -> (x/y=w531:dbl)
          }
          frame "One Ch PWA" {
            n315 = local read "No of samples"() -> (w534:i32)
            n316 = global read "PWAtasksGLOBAL.vi" "PWA Freq. (Hz)"() -> (w535:dbl)
            n317 = global write "PWAtasksGLOBAL.vi" "PWA No. of Samples"(w534) -> ()
            n318 = Divide(x=w534, y=w535) -> (x/y=w536:dbl)
          }
        }
        n319 = global read "Meas_global.vi" "Averaging time (min)"() -> (w525:dbl)
        n320 = Equal?(x=Setup."Run Program" ("setup"), y=w524) -> (x = y?=w522:bool)
        n321 = Equal?(x=Post_Process."Take New Data" ("Post Process"), y=w530) -> (x = y?=w526:bool)
        n322 = Compound Arithmetic op=AND(invert w518, w526, invert w520, invert w527, w522) -> (w528:bool)
        n323 = case shown="True" w528 {
          tunnel: w525 -> [_ w543]
          tunnel: w521 -> [_ w542]
          tunnel: w519 -> [_ w537]
          frame False {
          }
          frame True {
            n324 = global read "Meas_global.vi" "Board type"() -> (w540:T13)
            n325 = Equal?(x=w540, y=Board_Types."Simulate" ("Board type")) -> (x = y?=w539:bool)
            n326 = case shown="False" w539 {
              tunnel: w543 -> [w553 _]
              tunnel: w542 -> [w546 _]
              tunnel: [w545 1 ("No of Blocks")] -> w538
              tunnel: w537 -> [w544 _]
              frame False {
                n327 = Multiply(x=w553, y=60.0) -> (x*y=w551:dbl)
                n328 = global read "Meas_global.vi" "LDA data"() -> (w555:enum16{"No LDA data", "Take LDA data"})
                n329 = Equal?(x=enum16{"No LDA data", "Take LDA data"}."Take LDA data" ("LDA data"), y=w555) -> (x = y?=w549:bool)
                n330 = Divide(x=w551, y=w546) -> (x/y=w550:dbl)
                n331 = Round Toward +Infinity(x=w550) -> (ceil(x): smallest int >= x=w548:dbl)
                n332 = To Long Integer(number=w548) -> (32bit integer=w547:i32)
                n333 = case shown="\"No PWA Data\"" w544 {
                  tunnel: w549 -> [w559 _]
                  tunnel: w547 -> [w557 w560]
                  tunnel: [w556 w560] -> w545
                  frame "No PWA Data" {
                    n334 = Select(t=99999 ("No of Blocks"), s=w559, f=w557) -> (s? t:f=w556:i32)
                  }
                  frame "One Ch PWA" {
                  }
                }
              }
              frame True {
              }
            }
            n335 = global write "Meas_global.vi" "Requested No of blocks"(w538) -> ()
            n336 = local write "No of Blocks"(w538) -> ()
          }
        }
      }
      frame #15 {
        n337 = case shown="\"Run Program\"" w562 {
          frame "Run Program" {
            n338 = call "Read_calibration_files.vi"() -> ()  [unwired: 1 out]
            n339 = global write "Meas_global.vi" "Repeat Measurement?"(FALSE ("Repeat Measurement?")) -> ()
          }
          frame "Show Setup", Default {
          }
        }
      }
      frame #16 {
        n340 = global read "Meas_global.vi" "Raw data option"() -> (w567:enum16{"Save raw data", "Raw data not saved"})
        n341 = Get Date/Time In Seconds() -> (seconds since 1Jan1904=w568:timestamp)
        n342 = To Double Precision Float(number=w568) -> (double precision float=w565:dbl)
        n343 = global read "Meas_global.vi" "Post Process"() -> (w566:T5)
        n344 = case shown="\"Setup Front Panel\"" w569 {
          tunnel: w567 -> [w572 _ _ _]
          tunnel: w566 -> [w571 _ w604 w613]
          frame "Run Program" {
            n345 = case shown="\"Take New Data\"" w571 {
              tunnel: w572 -> [w573 _]
              frame "Take New Data" {
                n346 = case shown="\"Raw data not saved\"" w573 {
                  frame "Save raw data" {
                  }
                  frame "Raw data not saved" {
                    w581 = FALSE  # Lock File
                    w578 = FALSE  # advisory dialog? (display:T)
                    w577 = FALSE  # append to file? (new file:F)
                    n347 = global read "Meas_global.vi" "Remote control"() -> (w579:bool)
                    n348 = call "Create_setup_string.vi"() -> ("Setup String"=w582:string)  [unwired: 1 out]
                    n349 = case shown="False" w579 {
                      tunnel: ["Current_Setup.xls" ("Setup filename") w584] -> w574
                      frame False {
                      }
                      frame True {
                        n350 = local read "Setup filename"() -> (w584:string)
                      }
                    }
                    n351 = call "Add_length_to_string.vi"("String in"=w582) -> ("String out"=w580:string)
                    n352 = call "Setup_Filepath.vi"("Setup File Type"=Setup_Filetype."Measurement Setups", "Filename in"=w574) -> ("Filename Out"=w575:path)  [unwired: 1 out]
                    n353 = call "Write_Characters_To_File.vi"("file path (dialog if empty)"=w575, "advisory dialog? (display:T)"=w578, "character string"=w580, "append to file? (new file:F)"=w577, "Lock File"=w581) -> ()  [unwired: 4 out]
                  }
                }
              }
              frame "Post Process Raw Data File" {
              }
            }
          }
          frame "Save Current Setup" {
            n354 = stacked-sequence {
              seq-local: [w587 _] -> [_ w590]
              seq-local: [w586 _] -> [_ w589]
              frame #0 {
                w588 = FALSE  # Save New File?
                n355 = call "Save_current_setup.vi"("Save New File?"=w588, "Setup File Type"=Setup_Filetype."Measurement Setups") -> ("Cancelled?"=w586:bool, "Saved filepath"=w587:path)  [unwired: 2 out]
              }
              frame #1 {
                n356 = case shown="False" w589 {
                  tunnel: w590 -> [w596 _]
                  frame False {
                    w593 = "Initial Probe positions" ("File Label")
                    w601 = FALSE  # append to file? (new file:F)
                    w602 = FALSE  # advisory dialog? (display:T)
                    w603 = FALSE  # Lock File
                    n357 = call "Input_Instrument_Positions.vi"("Filepath to Save"=w596) -> ("Output string"=w595:string)  [unwired: 1 out]
                    n358 = call "Create_setup_string.vi"() -> ("Setup String"=w594:string)  [unwired: 1 out]
                    n359 = call "Get_string_subset.vi"("String to split"=w595, "File Label"=w593) -> ("Output string"=w592:string)  [unwired: 2 in, 1 out]
                    n360 = call "Replace_data_in_Label_str.vi"("New data string"=w592, "Input string"=w594, "Variable name"=w593) -> ("Appended string"=w591:string)
                    n361 = call "Replace_data_in_setup_string.vi"("New data string"="", "Input string"=w591, "Variable name"="Comments") -> ("Appended string"=w597:string)
                    n362 = call "Add_length_to_string.vi"("String in"=w597) -> ("String out"=w600:string)
                    n363 = call "Write_Characters_To_File.vi"("file path (dialog if empty)"=w596, "advisory dialog? (display:T)"=w602, "character string"=w600, "append to file? (new file:F)"=w601, "Lock File"=w603) -> ()  [unwired: 4 out]
                  }
                  frame True {
                  }
                }
              }
            }
          }
          frame "Show Setup" {
            n364 = case shown="\"Take New Data\"" w604 {
              frame "Take New Data" {
                w609 = FALSE  # append to file? (new file:F)
                w610 = FALSE  # advisory dialog? (display:T)
                w611 = FALSE  # Lock File
                n365 = call "Create_setup_string.vi"() -> ("Setup String"=w612:string)  [unwired: 1 out]
                n366 = call "Add_length_to_string.vi"("String in"=w612) -> ("String out"=w608:string)
                n367 = call "Setup_Filepath.vi"("Setup File Type"=Setup_Filetype."Measurement Setups", "Filename in"="Current_Setup.xls" ("Setup filename")) -> ("Filename Out"=w606:path)  [unwired: 1 out]
                n368 = call "Write_Characters_To_File.vi"("file path (dialog if empty)"=w606, "advisory dialog? (display:T)"=w610, "character string"=w608, "append to file? (new file:F)"=w609, "Lock File"=w611) -> ()  [unwired: 4 out]
              }
              frame "Post Process Raw Data File" {
              }
            }
          }
          frame "Setup Front Panel" {
            n369 = case shown="\"Take New Data\"" w613 {
              frame "Take New Data" {
                w618 = FALSE  # append to file? (new file:F)
                w619 = FALSE  # advisory dialog? (display:T)
                w620 = FALSE  # Lock File
                n370 = call "Create_setup_string.vi"() -> ("Setup String"=w621:string)  [unwired: 1 out]
                n371 = call "Add_length_to_string.vi"("String in"=w621) -> ("String out"=w617:string)
                n372 = call "Setup_Filepath.vi"("Setup File Type"=Setup_Filetype."Measurement Setups", "Filename in"="Current_Setup.xls" ("Setup filename")) -> ("Filename Out"=w615:path)  [unwired: 1 out]
                n373 = call "Write_Characters_To_File.vi"("file path (dialog if empty)"=w615, "advisory dialog? (display:T)"=w619, "character string"=w617, "append to file? (new file:F)"=w618, "Lock File"=w620) -> ()  [unwired: 4 out]
              }
              frame "Post Process Raw Data File" {
              }
            }
          }
        }
        n374 = call "Program_Active.vi"() -> ()  [unwired: 1 in]
        n375 = global write "Meas_global.vi" "Actual Measurement time (min)"(0.0 ("Max Measurement time (min)")) -> ()
        n376 = global write "Meas_global.vi" "Current Block No"(0 ("Current Block No")) -> ()
      }
      frame #17 {
        n377 = case shown="\"Setup Front Panel\", Default" w625 {
          tunnel: w622 -> [w627 _]
          tunnel: w624 -> [_ w814]
          tunnel: w623 -> [w626 _]
          frame "Run Program" {
            # "PWA"
            # "LDA"
            # "An"
            n378 = stacked-sequence {
              seq-local: [w635 _] -> [_ w657]
              seq-local: [w634 _] -> [_ w656]
              seq-local: [w633 _] -> [_ w655]
              seq-local: [w631 _] -> [_ w654]
              seq-local: [w629 _] -> [_ w651]
              seq-local: [w628 _] -> [_ w650]
              tunnel: w627 -> [_ w653]
              tunnel: w626 -> [_ w652]
              frame #0 {
                n379 = global read "Trav_pos_global.vi" "Dummy Measurement?"() -> (w630:bool)
                n380 = case shown="False" w630 {
                  tunnel: [w642 u16[][] [] ("LDA Binary output")] -> w635
                  tunnel: [w641 w644] -> w634
                  tunnel: [w640 dbl[][] [] ("Voltage output")] -> w633
                  tunnel: [w639 TRUE ("EOF?")] -> w632
                  tunnel: [w638 T15 {"Started"=0.0, "Ended"=0.0, "Analogue Frequency Hz"=1000.0} ("Block Timings")] -> w631
                  tunnel: [w637 w644] -> w629
                  tunnel: [w636 ""] -> w628
                  frame False {
                    n381 = call "Get_data.vi"() -> ("EOF? and Error status"=w639:bool, "Voltage output"=w640:dbl[][], "Analogue Binary"=w641:i16[][], "LDA Binary output"=w642:u16[][], "Block Timings"=w638:T15, "PWA Binary"=w637:i16[][], "Block Header"=w636:string)  [unwired: 5 out]
                  }
                  frame True {
                    w644 = i16[][] [] ("Analogue Binary")
                  }
                }
                n382 = case shown="True" w632 {
                  frame False {
                  }
                  frame True {
                    n383 = local write "No of Blocks"(1 ("No of Blocks")) -> ()
                  }
                }
              }
              frame #1 {
                n384 = while {
                  tunnel: w653 -> [w663]
                  shift-left: w654 -> [w664]
                  shift-right: [w665] -> _
                  shift-left: w655 -> [w669]
                  shift-right: [w672] -> _
                  shift-left: w656 -> [w670]
                  shift-right: [w673] -> _
                  shift-left: w657 -> [w671]
                  shift-right: [w674] -> _
                  tunnel: w652 -> [w662]
                  shift-right: [w661] -> _
                  shift-left: w651 -> [w660]
                  shift-right: [w659] -> _
                  shift-left: w650 -> [w658]
                  i -> [w666]
                  stop <- w675 continue-if-true
                  n385 = Increment(x=w666) -> (x+1=w676:i32)
                  n386 = stacked-sequence {
                    seq-local: [_ _ _ _ _ "Block average display control" _ _ _ _] -> [_ _ _ _ _ _ w771 _ _ _]
                    seq-local: [_ _ _ _ _ _ w768 _ _ _] -> [_ _ _ _ _ _ _ w782 _ _]
                    seq-local: [w712 _ _ _ _ _ _ _ _ _] -> [_ w718 _ _ w754 _ _ _ _ w812]
                    seq-local: [_ _ w723 _ _ _ _ _ _ _] -> [_ _ _ _ w752 _ _ _ _ _]
                    seq-local: [_ _ _ w744 _ _ _ _ _ _] -> [_ _ _ _ w753 _ _ _ _ _]
                    tunnel: w676 -> [w711 _ _ _ w756 w764 _ _ _ _]
                    tunnel: [_ _ _ _ _ _ _ _ _ w812] -> w675
                    tunnel: w666 -> [_ _ _ _ _ _ _ _ _ _]
                    tunnel: w671 -> [_ _ _ w742 _ _ _ _ _ _]
                    tunnel: w670 -> [_ _ _ w741 _ _ _ _ _ _]
                    tunnel: w669 -> [_ _ _ w748 _ _ _ _ _ _]
                    tunnel: "stop" -> [w714 _ _ _ _ _ _ _ _ _]
                    tunnel: "No of Blocks" -> [w713 _ _ _ _ _ _ _ _ _]
                    tunnel: w664 -> [_ _ _ w746 _ _ _ _ _ _]
                    tunnel: w663 -> [_ _ w722 w743 _ _ _ _ _ _]
                    tunnel: w662 -> [_ _ w724 _ _ _ _ _ _ _]
                    tunnel: w660 -> [_ _ _ w740 _ _ _ _ _ _]
                    tunnel: w658 -> [w710 _ _ _ _ _ _ _ _ _]
                    frame #0 {
                      n387 = global write "Plug_in_data_global.vi" "Block Header"(w710) -> ()
                      n388 = Less Or Equal?(x=w713, y=w711) -> (x <= y?=w716:bool)
                      n389 = Or(x=w714, y=w716) -> (x .or. y?=w715:bool)
                      n390 = global write "Meas_global.vi" "Current Block No"(w711) -> ()
                      n391 = Not(x=w715) -> (.not. x?=w712:bool)
                    }
                    frame #1 {
                      n392 = call "Program_Active.vi"() -> ()  [unwired: 1 in]
                      n393 = call "Text_without_format.vi"("Input string"="Comments") -> ("Output string"=w719:string)
                      n394 = global write "Meas_global.vi" "Position"("Position") -> ()
                      n395 = local write "Comments"(w719) -> ()
                      n396 = global write "Meas_global.vi" "Comments"(w719) -> ()
                      n397 = Not(x=w718) -> (.not. x?=w717:bool)
                      n398 = global write "Meas_global.vi" "Processing last block?"(w717) -> ()
                      n399 = global write "PWAtasksGLOBAL.vi" "STOP"(w717) -> ()
                    }
                    frame #2 {
                      n400 = case shown="False" w722 {
                        tunnel: w724 -> [w736 _]
                        tunnel: [w725 FALSE] -> w723
                        frame False {
                          w733 = 1.5  # To allow for overhead
                          n401 = Get Date/Time In Seconds() -> (seconds since 1Jan1904=w738:timestamp)
                          n402 = global read "Meas_global.vi" "Averaging time (min)"() -> (w732:dbl)
                          n403 = To Double Precision Float(number=w738) -> (double precision float=w737:dbl)
                          n404 = Subtract(x=w737, y=w736) -> (x-y=w735:dbl)
                          n405 = global read "Meas_global.vi" "LDA data"() -> (w729:enum16{"No LDA data", "Take LDA data"})
                          n406 = Divide(x=w735, y=60.0 ("To convert to minutes")) -> (x/y=w731:dbl)
                          n407 = Equal?(x=enum16{"No LDA data", "Take LDA data"}."Take LDA data" ("LDA data"), y=w729) -> (x = y?=w726:bool)
                          n408 = Multiply(x=w733, y=w732) -> (x*y=w730:dbl)
                          n409 = Greater?(x=w731, y=w730) -> (0:w727:bool)
                          n410 = And(x=w726, y=w727) -> (x .and. y?=w725:bool)
                        }
                        frame True {
                        }
                      }
                    }
                    frame #3 {
                      n411 = call "Process_data.vi"("PWA Binary"=w740, "Analogue Binary"=w741, "LDA Binary output"=w742, "Analogue volts"=w748, "Measurement top level?"=w743, "Block Timings"=w746) -> ("Vel stat display"=→"Statistics":string[][], "First Plot data"=→"First plot":cluster{"Xo":dbl, "Delta X":dbl, dbl[]}[], "Second Plot data"=→"2nd plot":cluster{"Xo":dbl, "Delta X":dbl, dbl[]}[], "Max Measurement time up"=w744:bool)
                    }
                    frame #4 {
                      n412 = global read "Meas_global.vi" "stop"() -> (w751:bool)
                      n413 = Compound Arithmetic op=OR(w751, w752, w753) -> (w750:bool)
                      n414 = And(x=w754, y=w750) -> (x .and. y?=w755:bool)
                      n415 = case shown="True" w755 {
                        tunnel: w756 -> [_ w757]
                        frame False {
                        }
                        frame True {
                          n416 = Increment(x=w757) -> (x+1=w758:i32)
                          n417 = local write "No of Blocks"(w758) -> ()
                        }
                      }
                    }
                    frame #5 {
                      n418 = global read "Meas_global.vi" "Actual Measurement time (min)"() -> (→"Measurement time (min)":dbl)
                      n419 = global read "Meas_global.vi" "Actual Sampling rate (Hz)"() -> (→"Actual Sampling freq":dbl)
                      n420 = call "Display_blocks.vi"("Block No"=w764, "Block average display"="Block average display control") -> ("u^4"=→"u^4":dbl[][], "u^3"=→"u^3":dbl[][], "uv"=→"uv":dbl[][], "u^2"=→"u^2" →"Array u^2":dbl[][], "U"=→"U" →"Array U":dbl[][])  [unwired: 4 out]
                    }
                    frame #6 {
                      n421 = global read "Meas_global.vi" "Analysis Info cluster"() -> (w770:T20[])
                      n422 = for {
                        tunnel: w771 -> [w776] mode=indexing
                        shift-right: [w772] -> w768
                        shift-left: u32[] [] -> [w773]
                        tunnel: w770 -> [w775] mode=indexing
                        n423 = Unbundle By Name(w776) -> ("Include"=w774:bool)
                        n424 = case shown="True" w774 {
                          tunnel: w775 -> [_ w781]
                          tunnel: w773 -> [w777 w779]
                          tunnel: [w777 w778] -> w772
                          frame False {
                          }
                          frame True {
                            n425 = Unbundle By Name(w781) -> ("Colour"=w780:u32)
                            n426 = Build Array (concatenate)(w779, w780) -> (w778:u32[])
                          }
                        }
                      }
                    }
                    frame #7 {
                      n427 = for {
                        tunnel: w782 -> [w783] mode=indexing
                        i -> [w784]
                        n428 = property on="U" class="WFGraph (strict)"("Active Plot"=w784, "Plot.Plot Color"=w783, "Plot.Fill/Point Color"=w783) -> ()  [unwired: 2 in, 2 out]
                        n429 = property on="u^3" class="WFGraph (strict)"("Active Plot"=w784, "Plot.Plot Color"=w783, "Plot.Fill/Point Color"=w783) -> ()  [unwired: 2 in, 2 out]
                        n430 = property on="u^4" class="WFGraph (strict)"("Active Plot"=w784, "Plot.Plot Color"=w783, "Plot.Fill/Point Color"=w783) -> ()  [unwired: 2 in, 2 out]
                        n431 = property on="u^2" class="WFGraph (strict)"("Active Plot"=w784, "Plot.Plot Color"=w783, "Plot.Fill/Point Color"=w783) -> ()  [unwired: 2 in, 2 out]
                      }
                    }
                    frame #8 {
                      n432 = case shown="True" "Pause" {
                        frame False {
                        }
                        frame True {
                          n433 = global read "Meas_global.vi" "Post Process"() -> (w786:T5)
                          n434 = case shown="\"Take New Data\"" w786 {
                            frame "Take New Data" {
                              n435 = call "Program_Active_Client.vi"("Mode"=enum16{"Program Active", "Traverse Level State"}."Program Active", "Time till next contact (Sec)"=12000.0, "Traverse level State"=Traverse_Level_State."Running") -> ()  [unwired: 3 out]
                              n436 = while {
                                i -> [w793]
                                stop <- w794 continue-if-true
                                n437 = Quotient & Remainder(x=w793, y=10) -> (x-y*floor(x/y)=w791:i32)  [unwired: 1 out]
                                n438 = Equal To 0?(x=w791) -> (x = 0?=w790:bool)
                                n439 = stacked-sequence {
                                seq-local: [_ w796 _ _] -> [_ _ w798 _]
                                tunnel: [_ w796 _ _] -> w794
                                tunnel: w790 -> [_ _ _ w800]
                                frame #0 {
                                "Pause message" <- "Measurement Program Paused!!!!" ("Pause message")
                                }
                                frame #1 {
                                n440 = global write "Trav_pos_global.vi" "Paused During Row?"(TRUE ("Paused During Row?")) -> ()
                                n441 = local read "Pause"() -> (w796:bool)
                                }
                                frame #2 {
                                n442 = property on="Pause message" class="Str"("Blinking"=w798, "Visible"=w798) -> ()  [unwired: 2 in, 2 out]
                                n443 = Wait Until Next ms Multiple(millisecond multiple=u32 1000) -> ()  [unwired: 1 out]
                                }
                                frame #3 {
                                n444 = case shown="False" w800 {
                                frame False {
                                }
                                frame True {
                                n445 = Current VI's Path() -> (path=w801:path)
                                n446 = call "Bring_to_front.vi"("path"=w801) -> ()
                                }
                                }
                                }
                                }
                              }
                            }
                            frame "Post Process Raw Data File" {
                              n447 = stacked-sequence {
                                seq-local: [_ w804 _ _] -> [_ _ _ w811]
                                frame #0 {
                                n448 = property on="PP next block" class="Bool (strict)"("Visible"=TRUE) -> ()  [unwired: 2 in, 2 out]
                                n449 = local write "PP next block"(FALSE ("PP next block")) -> ()
                                }
                                frame #1 {
                                n450 = while {
                                tunnel: [w808] -> w804
                                stop <- w805 stop-if-true
                                n451 = local read "stop"() -> (w808:bool)
                                n452 = local read "Pause"() -> (w806:bool)
                                n453 = Compound Arithmetic op=OR(w808, "PP next block", invert w806) -> (w805:bool)
                                n454 = case shown="False" w805 {
                                frame False {
                                n455 = Wait (ms)(milliseconds to wait=u32 200) -> ()  [unwired: 1 out]
                                }
                                frame True {
                                }
                                }
                                }
                                }
                                frame #2 {
                                n456 = property on="PP next block" class="Bool (strict)"("Visible"=FALSE) -> ()  [unwired: 2 in, 2 out]
                                }
                                frame #3 {
                                n457 = Stop(stop? (T)=w811) -> ()
                                }
                              }
                            }
                          }
                        }
                      }
                    }
                    frame #9 {
                      n458 = global read "Meas_global.vi" "Diagnostic info"() -> (→"BSA Diagnostic info":string[][])
                    }
                  }
                  n459 = stacked-sequence {
                    seq-local: [w678 _ _] -> [_ w688 _]
                    seq-local: [_ w687 _] -> [_ _ w708]
                    tunnel: [_ w691 _] -> w674
                    tunnel: [_ w690 _] -> w673
                    tunnel: [_ w689 _] -> w672
                    tunnel: "No of Blocks" -> [w683 _ _]
                    tunnel: "stop" -> [w681 _ _]
                    tunnel: w666 -> [w679 _ w707]
                    tunnel: [_ w686 _] -> w665
                    tunnel: [_ w685 _] -> w661
                    tunnel: [_ w684 _] -> w659
                    frame #0 {
                      n460 = Increment(x=w679) -> (x+1=w677:i32)
                      "Current Block No" <- w677
                      n461 = Less Or Equal?(x=w683, y=w677) -> (x <= y?=w682:bool)
                      n462 = Or(x=w682, y=w681) -> (x .or. y?=w680:bool)
                      n463 = Not(x=w680) -> (.not. x?=w678:bool)
                      n464 = global write "Meas_global.vi" "Current Block No"(w677) -> ()
                    }
                    frame #1 {
                      n465 = case shown="True" w688 {
                        tunnel: [u16[][] [] ("LDA Binary output") w704] -> w691
                        tunnel: [w693 w703] -> w690
                        tunnel: [dbl[][] [] ("Voltage output") w702] -> w689
                        tunnel: [FALSE ("EOF?") w701] -> w687
                        tunnel: [T15 {"Started"=0.0, "Ended"=0.0, "Analogue Frequency Hz"=200.0} ("Block Timings") w700] -> w686
                        tunnel: [w693 w699] -> w685
                        tunnel: ["" w698] -> w684
                        frame False {
                          w693 = i16[][] [] ("Analogue Binary")
                        }
                        frame True {
                          n466 = call "Get_data.vi"() -> ("EOF? and Error status"=w701:bool, "Voltage output"=w702:dbl[][], "Analogue Binary"=w703:i16[][], "LDA Binary output"=w704:u16[][], "Block Timings"=w700:T15, "PWA Binary"=w699:i16[][], "Block Header"=w698:string)  [unwired: 5 out]
                        }
                      }
                    }
                    frame #2 {
                      n467 = Increment(x=w707) -> (x+1=w705:i32)
                      n468 = Increment(x=w705) -> (x+1=w706:i32)
                      n469 = case shown="True" w708 {
                        tunnel: w706 -> [_ w709]
                        frame False {
                        }
                        frame True {
                          n470 = local write "No of Blocks"(w709) -> ()
                        }
                      }
                    }
                  }
                }
              }
            }
          }
          frame "Setup Front Panel", Default {
            n471 = stacked-sequence {
              seq-local: [w815 _ _ _ _ _ _] -> [_ _ _ _ _ w889 _]
              seq-local: [_ w821 _ _ _ _ _] -> [_ _ _ _ _ w888 _]
              seq-local: [_ _ _ w852 _ _ _] -> [_ _ _ _ _ w887 _]
              seq-local: [_ _ _ _ w865 _ _] -> [_ _ _ _ _ w885 _]
              seq-local: [_ w820 _ _ _ _ _] -> [_ _ _ _ _ _ w902]
              seq-local: [_ _ w846 _ _ _ _] -> [_ _ _ _ _ w884 _]
              tunnel: w814 -> [_ w822 _ _ _ _ _]
              frame #0 {
                n472 = Build Array("Name", "Channel", "High limit", "Low limit") -> (w815:string[])
              }
              frame #1 {
                n473 = global read "Meas_global.vi" "LDA data"() -> (w820:enum16{"No LDA data", "Take LDA data"})
                n474 = case shown="\"Take LDA data\"" w820 {
                  tunnel: w822 -> [_ w833]
                  tunnel: [string[][] [] w830] -> w821
                  frame "No LDA data" {
                  }
                  frame "Take LDA data" {
                    n475 = case shown="\"2D\"" w833 {
                      tunnel: [string[] [] w839] -> w831
                      frame "1D" {
                      }
                      frame "2D" {
                        n476 = global read "LDA_meas_global_2.vi" "Max Vel BSA2"() -> (w838:dbl)
                        n477 = global read "LDA_meas_global_2.vi" "Min Vel BSA2"() -> (w837:dbl)
                        n478 = global read "LDA_meas_global_2.vi" "Vel Comp BSA2"() -> (w840:string)
                        n479 = Format Into String(format string="%.1f m/s" ("Format String"), w837) -> (resulting string=w845:string)  [unwired: 2 in, 1 out]
                        n480 = Format Into String(format string="%.1f m/s" ("Format String"), w838) -> (resulting string=w844:string)  [unwired: 2 in, 1 out]
                        n481 = Build Array("LDA", w840, w844, w845) -> (w839:string[])
                      }
                    }
                    n482 = global read "LDA_meas_global_1.vi" "Max Vel BSA1"() -> (w825:dbl)
                    n483 = global read "LDA_meas_global_1.vi" "Min Vel BSA1"() -> (w824:dbl)
                    n484 = global read "LDA_meas_global_1.vi" "Vel Comp BSA1"() -> (w834:string)
                    n485 = Format Into String(format string="%.1f m/s" ("Format String"), w824) -> (resulting string=w826:string)  [unwired: 2 in, 1 out]
                    n486 = Format Into String(format string="%.1f m/s" ("Format String"), w825) -> (resulting string=w827:string)  [unwired: 2 in, 1 out]
                    n487 = Build Array("LDA", w834, w827, w826) -> (w832:string[])
                    n488 = Build Array(w832, w831) -> (w830:string[][])
                  }
                }
              }
              frame #2 {
                n489 = global read "Meas_global.vi" "PWA Data"() -> (w847:T31)
                n490 = case shown="\"One Ch PWA\"" w847 {
                  tunnel: [string[][] [] w849] -> w846
                  frame "No PWA Data" {
                  }
                  frame "One Ch PWA" {
                    n491 = Build Array("PWA") -> (w850:string[])
                    n492 = Build Array(w850) -> (w849:string[][])
                  }
                }
              }
              frame #3 {
                n493 = global read "Meas_global.vi" "Ch & spans"() -> (w853:T26[])
                n494 = for {
                  tunnel: w853 -> [w864] mode=indexing
                  tunnel: [w860] -> w852 mode=indexing
                  n495 = Unbundle By Name(w864) -> ("Var name"=w863:string, "Ch No"=w862:i16, "high limit (10V)"=w857:sgl, "low limit (-10V)"=w856:sgl)
                  n496 = Format Into String(format string="%.1f Volts" ("Format String"), w857) -> (resulting string=w855:string)  [unwired: 2 in, 1 out]
                  n497 = Format Into String(format string="%.1f Volts" ("Format String"), w856) -> (resulting string=w854:string)  [unwired: 2 in, 1 out]
                  n498 = Number To Decimal String(number=w862) -> (decimal integer string=w861:string)  [unwired: 1 out]
                  n499 = Build Array(w863, w861, w855, w854) -> (w860:string[])
                }
              }
              frame #4 {
                n500 = global read "Meas_global.vi" "Analysis Info cluster"() -> (w873:T20[])
                n501 = for {
                  tunnel: w873 -> [w883] mode=indexing
                  tunnel: [w882] -> w871 mode=indexing
                  n502 = Unbundle By Name(w883) -> ("Inst name"=w882:string)
                }
                n503 = global read "Meas_global.vi" "correlate"() -> (w872:i32[][])
                n504 = for {
                  tunnel: w872 -> [w878] mode=indexing
                  tunnel: w871 -> [w877]
                  tunnel: "Correlating" -> [w876]
                  tunnel: [w874] -> w866 mode=indexing
                  n505 = for {
                    tunnel: w878 -> [w881] mode=indexing
                    tunnel: w877 -> [w880]
                    tunnel: [w879] -> w875 mode=indexing
                    n506 = Index Array(array=w880, index=w881) -> (element=w879:string)
                  }
                  n507 = Build Array (concatenate)(w876, w875) -> (w874:string[])
                }
                n508 = Initialize Array("", 5 ("Dimension Size")) -> (w867:string[])
                n509 = Build Array (concatenate)(w867, w866) -> (w865:string[][])
              }
              frame #5 {
                n510 = Build Array (concatenate)(w889, w888, w884, w887, w885) -> (w886:string[][])
                n511 = local write "Statistics"(w886) -> ()
              }
              frame #6 {
                n512 = global read "Meas_global.vi" "Board type"() -> (w900:T13)
                n513 = global read "Meas_global.vi" "Continuous time trace?"() -> (w901:bool)
                n514 = Equal?(x=w900, y=Board_Types."ADC488" ("Board type")) -> (x = y?=w898:bool)
                n515 = case shown="\"Take LDA data\"" w902 {
                  tunnel: w898 -> [_ w906]
                  tunnel: [string[] [] w905] -> w894
                  frame "No LDA data" {
                  }
                  frame "Take LDA data" {
                    n516 = global read "Meas_global.vi" "Synchronise with LDA"() -> (w911:bool)
                    n517 = global read "Meas_global.vi" "Ch & spans"() -> (w914:T26[])
                    n518 = global read "LDA_meas_global_1.vi" "Probe Configuration"() -> (w904:string)
                    n519 = Array Size(array=w914) -> (size(s)=w913:i32)
                    n520 = Greater Than 0?(x=w913) -> (x > 0?=w912:bool)
                    n521 = Compound Arithmetic op=AND(w911, w906, w912) -> (w910:bool)
                    n522 = Select(t="Synchronised with LDA", s=w910, f="") -> (s? t:f=w907:string)
                    n523 = Build Array(w904, w907) -> (w905:string[])
                  }
                }
                n524 = Compound Arithmetic op=AND(w898, w901) -> (w895:bool)
                n525 = Select(t="Continuous Time Trace", s=w895, f="") -> (s? t:f=w893:string)
                n526 = Build Array (concatenate)(w894, w893) -> (w892:string[])
                n527 = Build Array(w892) -> (w891:string[][])
                n528 = Transpose 2D Array(2D array=w891) -> (transposed array=w890:string[][])
                n529 = local write "BSA Diagnostic info"(w890) -> ()
              }
            }
          }
        }
      }
      frame #18 {
        n530 = local read "File"() -> (w932:T9)
        n531 = Equal?(x=Setup."Run Program" ("setup"), y=w933) -> (x = y?=w930:bool)
        n532 = Not Equal?(x=w932, y=Save_Data."Save No Data" ("File")) -> (x != y?=w931:bool)
        n533 = global read "Meas_global.vi" "Repeat Measurement?"() -> (w915:bool)
        n534 = Compound Arithmetic op=AND(invert w915, w930, w931) -> (w929:bool)
        n535 = Get Date/Time In Seconds() -> (seconds since 1Jan1904=w926:timestamp)
        n536 = To Double Precision Float(number=w926) -> (double precision float=w918:dbl)
        n537 = local read "Setup filename"() -> (w927:string)
        n538 = global read "Trav_pos_global.vi" "Meas Setup Number"() -> (w924:i32)
        n539 = global read "Meas_global.vi" "Board type"() -> (w922:T13)
        n540 = Greater Than 0?(x=w924) -> (x > 0?=w920:bool)
        n541 = Equal?(x=w922, y=Board_Types."Simulate" ("Board type")) -> (x = y?=w921:bool)
        n542 = And(x=w920, y=w921) -> (x .and. y?=w919:bool)
        n543 = case shown="True" w919 {
          tunnel: w918 -> [_ w937]
          tunnel: [w934 w935] -> w917
          tunnel: w916 -> [w934 _]
          frame False {
          }
          frame True {
            n544 = global read "Trav_pos_global.vi" "Current Row"() -> (w940:T17)
            n545 = Unbundle By Name(w940) -> ("Averaging time (min)"=w938:dbl)
            n546 = Multiply(x=60.0 ("y"), y=w938) -> (x*y=w936:dbl)
            n547 = Subtract(x=w937, y=w936) -> (x-y=w935:dbl)
          }
        }
        n548 = case shown="True" w929 {
          tunnel: w932 -> [_ _]
          tunnel: w918 -> [w943 w995]
          tunnel: w927 -> [w942 w994]
          tunnel: w917 -> [w941 w993]
          frame True {
            n549 = stacked-sequence {
              seq-local: [_ w947 _ _ _] -> [_ _ w953 _ _]
              seq-local: [_ _ _ w966 _] -> [_ _ _ _ w986]
              tunnel: w943 -> [w946 _ _ _ _]
              tunnel: w942 -> [w945 _ _ _ _]
              tunnel: w941 -> [w944 _ _ _ _]
              frame #0 {
                n550 = call "Write_Results_file.vi"("Experiment start time"=w944, "Experiment End time"=w946, "Setup filename"=w945) -> ()  [unwired: 4 out]
              }
              frame #1 {
                n551 = global read "Meas_global.vi" "Second Graph"() -> (w951:T3)
                n552 = global read "Meas_global.vi" "First Graph"() -> (w952:T3)
                n553 = Unbundle By Name(w951) -> ("Save graph"=w949:u16)
                n554 = Unbundle By Name(w952) -> ("Save graph"=w950:u16)
                n555 = Add(x=w950, y=w949) -> (x+y=w948:u16)
                n556 = Not Equal To 0?(x=w948) -> (x != 0?=w947:bool)
              }
              frame #2 {
                n557 = case shown="True" w953 {
                  frame False {
                  }
                  frame True {
                    n558 = stacked-sequence {
                      tunnel: "Show Smoth" -> [w957 w958]
                      frame #0 {
                        n559 = local read "First plot"() -> (w956:cluster{"Xo":dbl, "Delta X":dbl, dbl[]}[])
                        n560 = local read "2nd plot"() -> (w955:cluster{"Xo":dbl, "Delta X":dbl, dbl[]}[])
                        n561 = call "Save_plot_routine.vi"("Show Smooth"=w957, "First Plot data"=w956, "Second Plot data"=w955) -> ()  [unwired: 1 in, 3 out]
                      }
                      frame #1 {
                        n562 = case shown="True" w958 {
                          frame False {
                          }
                          frame True {
                            n563 = Open VI Reference(vi path="Measurement.vi") -> (vi reference=w964:refnum<vi>, error out=w960:errorcluster)  [unwired: 1 in, 4 out]
                            n564 = local write "Show Smoth"(FALSE ("Show Smoth")) -> ()
                            n565 = property class="VI"(reference=w964, error in=w960, "Front Panel Window:Is Frontmost"=TRUE) -> (reference out=w962:refnum<vi>, error out=w961:errorcluster)
                            n566 = Close Reference(reference=w962, error in (no error)=w961) -> ()  [unwired: 1 out]
                          }
                        }
                      }
                    }
                  }
                }
              }
              frame #3 {
                w971 = FALSE  # Empty list
                n567 = global read "Meas_global.vi" "Raw data file"() -> (w970:path)
                n568 = global read "Trav_pos_global.vi" "Top level setup filename"() -> (w968:path)
                n569 = global read "Meas_global.vi" "Start Time of experiment"() -> (w967:dbl)
                n570 = Strip Path(path=w970) -> (stripped path=w966:path)  [unwired: 1 out]
                n571 = Empty String/Path?(string/path=w968) -> (empty?=w969:bool)
                n572 = case shown="False" w969 {
                  tunnel: w968 -> [w985 _]
                  tunnel: w966 -> [w983 _]
                  tunnel: w967 -> [w981 _]
                  frame False {
                    n573 = call "Sec_to_date_filename.vi"("seconds"=w981) -> ("Day"=w980:string, "Time"=w979:string)  [unwired: 2 out]
                    n574 = Format Into String(format string="Cmd_%s_%s.xls", w980, w979) -> (resulting string=w977:string)  [unwired: 2 in, 1 out]
                    n575 = call "Fast_string_Replace.vi"("Replace match with:"="-", "Input String"=w977, "regular expression"=":") -> ("Output String"=w974:string)  [unwired: 2 out]
                    n576 = call "Fast_string_Replace.vi"("Replace match with:"="", "Input String"=w974, "regular expression"=" ") -> ("Output String"=w972:string)  [unwired: 2 out]
                    n577 = Build Path(base path=w983, name or relative path=w972) -> (appended path=w982:path)
                    n578 = Copy(10:w982, 11:w985) -> ()  [unwired: 1 in, 5 out]
                  }
                  frame True {
                  }
                }
                n579 = call "Remember_RD_Folders.vi"("Empty list"=w971, "Folders to Remember"=w966) -> ()  [unwired: 1 out]
              }
              frame #4 {
                n580 = global read "Meas_global.vi" "LDA data"() -> (w987:enum16{"No LDA data", "Take LDA data"})
                n581 = case shown="\"Take LDA data\"" w987 {
                  tunnel: w986 -> [_ w991]
                  frame "No LDA data" {
                  }
                  frame "Take LDA data" {
                    w989 = "LDA_Probe_Orientation.txt" ("name or relative path")
                    n582 = call "Setup_Filepath.vi"("Setup File Type"=Setup_Filetype."General", "Filename in"=w989) -> ("Filename Out"=w988:path)  [unwired: 1 out]
                    n583 = Build Path(base path=w991, name or relative path=w989) -> (appended path=w992:path)
                    n584 = Copy(10:w992, 11:w988) -> ()  [unwired: 1 in, 5 out]
                  }
                }
              }
            }
          }
          frame False {
            n585 = global read "Meas_global.vi" "Raw data option"() -> (w996:enum16{"Save raw data", "Raw data not saved"})
            n586 = case shown="\"Save raw data\"" w996 {
              tunnel: w993 -> [w999 _]
              tunnel: w995 -> [w998 _]
              tunnel: w994 -> [w997 _]
              frame "Save raw data" {
                n587 = stacked-sequence {
                  tunnel: w999 -> [_ w1008]
                  tunnel: w998 -> [_ w1007]
                  tunnel: w997 -> [_ w1005]
                  frame #0 {
                    n588 = global read "Meas_global.vi" "Current Block No"() -> (w1000:i32)
                    n589 = global write "Meas_global.vi" "Requested No of blocks"(w1000) -> ()
                  }
                  frame #1 {
                    n590 = call "Create_Raw_data_file.vi"("No of averages"=1, "End time"=w1007, "Start time"=w1008, "Setup filename"=w1005) -> ("Values"=w1003:string[][], "Column headers"=w1004:string[])  [unwired: 2 out]
                    n591 = Index Array(array=w1003, index (row)=0) -> (element=w1001:string[])  [unwired: 1 in]
                    n592 = global write "Dynamic_call_global.ph.vi" "Plug in values"(w1001) -> ()
                    n593 = global write "Dynamic_call_global.ph.vi" "Plug in titles"(w1004) -> ()
                  }
                }
              }
              frame "Raw data not saved" {
              }
            }
          }
        }
      }
      frame #19 {
        n594 = stacked-sequence {
          seq-local: [w1015 _] -> [_ w1024]
          seq-local: [w1011 _] -> [_ w1023]
          tunnel: w1009 -> [w1022 _]
          frame #0 {
            n595 = global read "Meas_global.vi" "Raw data file"() -> (w1013:path)
            n596 = global read "Meas_global.vi" "Raw data option"() -> (w1021:enum16{"Save raw data", "Raw data not saved"})
            n597 = Equal?(x=Setup."Run Program" ("setup"), y=w1022) -> (x = y?=w1017:bool)
            n598 = Strip Path(path=w1013) -> (stripped path=w1012:path)  [unwired: 1 out]
            n599 = Equal?(x=w1021, y=enum16{"Save raw data", "Raw data not saved"}."Save raw data" ("Raw data option")) -> (x = y?=w1016:bool)
            n600 = Build Path(base path=w1012, name or relative path="VI_History.xls") -> (appended path=w1011:path)
            n601 = call "Does_file_exist_(simple).vi"("Pathname"=w1011) -> ("exists?"=w1019:bool)
            n602 = Not(x=w1019) -> (.not. x?=w1018:bool)
            n603 = Compound Arithmetic op=AND(w1018, w1017, w1016) -> (w1015:bool)
          }
          frame #1 {
            n604 = case shown="True" w1024 {
              tunnel: w1023 -> [_ w1031]
              frame False {
              }
              frame True {
                w1025 = FALSE  # Lock File
                n605 = global read "Meas_global.vi" "Prog's last revision date"() -> (w1028:u32)
                n606 = Get Date/Time String(date format (0)=enum16{"short", "long", "abbreviated"}."abbreviated", seconds (now)=w1028) -> (date string=w1027:string)  [unwired: 2 out]
                n607 = call "Characters_to_string.vi"("Characters to write"=w1027, "Label for characters"="Prog's last revision date") -> ("Output string"=w1033:string)
                n608 = call "Date_and_Time_to_string.vi"() -> ("Date and time (spreadsheet)"=w1034:string)
                n609 = call "Get_mod_dates.vi"() -> ("error out"=w1032:errorcluster, "Output string"=w1026:string)  [unwired: 1 in, 3 out]
                n610 = call "EnFlo_Error_Handler.vi"("error in (no error)"=w1032) -> ()  [unwired: 2 in, 3 out]
                n611 = Concatenate Strings(w1034, w1033, w1026) -> (w1030:string)
                n612 = call "Write_Characters_To_File.vi"("file path (dialog if empty)"=w1031, "character string"=w1030, "Lock File"=w1025) -> ()  [unwired: 2 in, 4 out]
              }
            }
          }
        }
      }
      frame #20 {
        w1038 = FALSE ("Remote control")
        n613 = local read "Correlate?"() -> (w1040:T6)
        n614 = case shown="\"Run Program\"" w1037 {
          tunnel: w1037 -> [w1044 _ _ _]
          tunnel: [w1044 w1061 w1062 w1063] -> w1036
          frame "Run Program" {
            n615 = global read "Meas_global.vi" "Velocity Cluster Array"() -> (w1043:T27[])
            n616 = Array Size(array=w1043) -> (size(s)=w1042:i32)
            n617 = Decrement(x=w1042) -> (x-1=w1041:i32)
            n618 = while {
              tunnel: w1043 -> [w1059] mode=indexing
              tunnel: w1041 -> [w1050]
              i -> [w1051]
              stop <- w1048 continue-if-true
              w1056 = "Pitot ("
              n619 = Unbundle By Name(w1059) -> ("U"=w1045:dbl, "Name"=w1055:string)
              n620 = String Length(string=w1056) -> (length=w1058:i32)
              n621 = String Subset(string=w1055, length (rest)=w1058) -> (substring=w1057:string)  [unwired: 1 out]
              n622 = Equal?(x=w1057, y=w1056) -> (x = y?=w1052:bool)
              n623 = call "Match_Pat_Case_In.vi"("String to match"="ref", "String"=w1055) -> ("offset past match"=w1053:i32)  [unwired: 1 in, 3 out]
              n624 = Greater Or Equal To 0?(x=w1053) -> (x >= 0?=w1047:bool)
              n625 = Less?(x=w1051, y=w1050) -> (x < y?=w1049:bool)
              n626 = And(x=w1047, y=w1052) -> (x .and. y?=w1046:bool)
              n627 = case shown="True" w1046 {
                tunnel: w1045 -> [_ w1060]
                frame False {
                }
                frame True {
                  n628 = call "Log_Reference_Velocity.vi"("Measured Velocity"=w1060) -> ()  [unwired: 1 out]
                }
              }
              n629 = Compound Arithmetic op=AND(invert w1046, w1049) -> (w1048:bool)
            }
          }
          frame "Show Setup" {
            w1061 = Setup."Run Program"  # setup
          }
          frame "Save Current Setup" {
            w1062 = Setup."Run Program"  # setup
          }
          frame "Setup Front Panel" {
            w1063 = Setup."Run Program"  # setup
          }
        }
        n630 = case shown="\"Correlate without activating panel\"" w1040 {
          tunnel: [T6."Cross correlation off" T6."Correlate without activating panel" T6."Correlate without activating panel"] -> w1039
          frame "Cross correlation off" {
          }
          frame "Show correlation panel" {
          }
          frame "Correlate without activating panel" {
          }
        }
        n631 = local write "Correlate?"(w1039) -> ()
        n632 = global write "Meas_global.vi" "Remote control"(w1038) -> ()
        n633 = global write "Dynamic_call_global.ph.vi" "Acquisition Interlock"(w1038) -> ()
        n634 = call "Program_Active.vi"() -> ()  [unwired: 1 in]
        n635 = local write "setup"(w1036) -> ()
      }
      frame #21 {
        w1071 = FALSE  # Dialog Box (T)
        n636 = global read "Meas_global.vi" "Over/Under string"() -> (w1069:string)
        n637 = Empty String/Path?(string/path=w1069) -> (empty?=w1068:bool)
        n638 = Not(x=w1068) -> (.not. x?=w1067:bool)
        n639 = Bundle By Name(cluster=errorcluster {"status"=FALSE, "code"=0, "source"=""} ("error in (no error)"), "source"=w1069, "status"=w1067) -> (w1072:errorcluster)
        n640 = call "EnFlo_Error_Handler.vi"("error in (no error)"=w1072, "Error Type"="Signal Clipping", "Dialog Box (T)"=w1071) -> ()  [unwired: 3 out]
      }
      frame #22 {
        w1076 = string[] [] ("Per Block Plug Ins Extra")
        n641 = Empty String/Path?(string/path=w1080) -> (empty?=w1079:bool)
        n642 = global read "Dynamic_call_global.ph.vi" "Final Plug Ins"() -> (w1081:string[])
        n643 = case shown="True" w1079 {
          tunnel: w1080 -> [w1093 _]
          frame False {
            n644 = local read "Comments"() -> (w1092:string)
            n645 = call "Fast_string_Replace.vi"("Replace match with:"="", "Input String"=w1092, "regular expression"=w1093) -> ("Output String"=w1091:string)  [unwired: 2 out]
            n646 = local write "Comments"(w1091) -> ()
          }
          frame True {
          }
        }
        n647 = call "Plug_in_Directories.vi"() -> ("Final"=w1077:path)  [unwired: 3 out]
        n648 = for {
          tunnel: w1081 -> [w1096] mode=indexing
          tunnel: w1077 -> [w1095]
          w1099 = FALSE  # Dialog Box (T)
          n649 = Build Path(base path=w1095, name or relative path=w1096) -> (appended path=w1094:path)
          n650 = global read "Dynamic_call_global.ph.vi" "Plug in"() -> (w1104:refnum<vi>)
          n651 = Open VI Reference(type specifier VI Refnum (for type only)=w1104, vi path=w1094) -> (vi reference=w1103:refnum<vi>, error out=w1102:errorcluster)  [unwired: 2 in, 2 out]
          n652 = call-by-ref "?"(reference=w1103, error in=w1102) -> (reference out=w1100:refnum<vi>, error out=w1101:errorcluster)  [unwired: 6 in, 2 out]
          n653 = Close Reference(reference=w1100, error in (no error)=w1101) -> (error out=w1097:errorcluster)
          n654 = call "EnFlo_Error_Handler.vi"("error in (no error)"=w1097, "Error Type"="Running Final Plug In", "Dialog Box (T)"=w1099) -> ()  [unwired: 3 out]
        }
        n655 = global read "Meas_global.vi" "Repeat Measurement?"() -> (w1078:bool)
        n656 = case shown="False" w1078 {
          tunnel: w1075 -> [_ w1089]
          tunnel: [FALSE w1084] -> w1074
          frame False {
            n657 = global write "Trav_pos_global.vi" "Present Probe Positions"(T7 [] ("Present Probe Positions")) -> ()
          }
          frame True {
            n658 = global read "Meas_global.vi" "Post Process"() -> (w1087:T5)
            n659 = Equal To 0?(x=w1089) -> (x = 0?=w1085:bool)
            n660 = Equal?(x=w1087, y=Post_Process."Post Process Raw Data File" ("Post Process")) -> (x = y?=w1086:bool)
            n661 = And(x=w1086, y=w1085) -> (x .and. y?=w1084:bool)
          }
        }
        n662 = global write "Dynamic_call_global.ph.vi" "Per Block Plug Ins Extra"(w1076) -> ()
        n663 = global write "Dynamic_call_global.ph.vi" "Initial Plug Ins Extra"(w1076) -> ()
      }
      frame #23 {
        n664 = global read "Meas_global.vi" "Post Process"() -> (w1111:T5)
        n665 = local read "stop"() -> (w1117:bool)
        n666 = Equal?(x=w1112, y=Setup."Run Program" ("setup")) -> (x = y?=w1108:bool)
        n667 = Equal?(x=w1111, y=Post_Process."Take New Data" ("Post Process")) -> (x = y?=w1109:bool)
        n668 = And(x=w1108, y=w1109) -> (x .and. y?=w1107:bool)
        n669 = case shown="False" w1117 {
          tunnel: [Multi_Run_Status."Continue" ("Status Out") Multi_Run_Status."Terminate Run" ("Status Out")] -> w1115
          frame False {
          }
          frame True {
            n670 = local write "stop"(FALSE) -> ()
          }
        }
        n671 = case shown="True" w1107 {
          tunnel: w1115 -> [w1118 w1121]
          tunnel: [w1118 w1123] -> w1114
          frame False {
          }
          frame True {
            n672 = local read "Raw data file"() -> (w1122:path)
            n673 = Path to Array of Strings(0:w1122) -> (2:w1124:string[])  [unwired: 1 out]
            n674 = Index Array(array=w1124, index=0 ("Index")) -> (element=w1120:string)
            n675 = Build Array(w1120) -> (w1119:string[])
            n676 = for {
              tunnel: w1119 -> [w1128] mode=indexing
              shift-right: [w1126] -> w1123
              shift-left: w1121 -> [w1127]
              n677 = call "Warn_on_low_HD_space.vi"("Status In"=w1127, "HD name"=w1128) -> ("Status Out"=w1126:T4)  [unwired: 6 out]
            }
          }
        }
        "Status Out" <- w1114
        n678 = global write "Trav_pos_global.vi" "Dummy Measurement?"(FALSE ("Dummy Measurement?")) -> ()
        n679 = global write "Plug_in_data_global.vi" "Server Channels to log"(string[] [] ("Server Channels to log")) -> ()
        n680 = global write "Meas_global.vi" "Extra Comments"("") -> ()
      }
    }
  }
